vi "PPMS Interface_dev_IVdynamic.vi"() -> ()   [LabVIEW 2020]
uses:
  <vilib>/Analysis/1siggen.llb/Ramp Pattern by Samples.vi
  <vilib>/Utility/file.llb/Write Delimited Spreadsheet (string).vi
  <vilib>/Utility/file.llb/Write Delimited Spreadsheet (DBL).vi
  <vilib>/Analysis/NI_AALBase.lvlib
panel:
  in  "AC IV Path":path=path "C:/Users/QDUser/Desktop/LabVIEW Programs/PPMS Interface/lib/Measure IV AC.vi"
  out "IV Data":dbl[][](array[numeric])
  in  "DC IV Path":path=path "C:/Users/QDUser/Desktop/LabVIEW Programs/PPMS Interface/lib/Measure IV DC.vi"
  in  "scan_npts":i16
  out "scan_points":dbl[](array[numeric])
  out "scan_RATE":dbl=20.0
  out "scan_counter":i16=1000
  out "scan_head":i32=55
  out "scan_new":bool caption="Scan New"
  out "scan_env":string="MEASURE"
  out "Seq Line Now":i32=55
  out "AC Flag":bool caption="AC Current"
  in  "Filetype":u16(ring)=2 items=[".xlsx", ".txt", ".csv"]
  out "Wait Done":dbl=10.0
  in  "Measurement setup tabs":enum32{"DC Setup", "AC Setup", "I-V Setup"}(tab)=enum."AC Setup"
  in  "DC Pulse":bool=TRUE caption="Current Pulsing"
  in  "Channel 2":bool
  in  "Channel 1":bool=TRUE
  in  "Current Amplitude":string="1e-4"
  in  "Time Period (s)":string="3"
  in  "Tpad(ms)":i32=200
  in  "Voltmeter Range (V)":string="0.01"
  in  "NPLC":string="1"
  in  "Voltmeter Buffer Size":string="62"
  in  "Voltmeter 2 Address":string="8"
  in  "Voltmeter 1 Address":string="7"
  in  "6221 Address":string="12"
  in  "Configure DC System":bool
  in  "6221 Address 2":string="12" caption="6221 Address"
  in  "Current Amplitude 2":string="1e-4" caption="Current \nAmplitude"
  in  "Ch2 Enable":bool
  in  "Ch1 Enable":bool=TRUE
  in  "Buffer Data":enum16{"X", "XY", "RT", "XYRT"}(ring)=enum."RT"
  in  "Rate decimation":i32=2
  in  "SR860 Ch2 Address":string="5"
  in  "SR860 Ch1 Address":string="4"
  in  "Frequency":string="1711"
  in  "Filter BW":T1(ring)=enum."100ms"
  in  "Ch1 Harmonic":T2(ring)
  in  "Buffer Size (kB)":i32=2
  in  "Configure AC System":bool
  in  "Buffer Offset (kb)":string="0"
  in  "Ch2 Harmonic":T2(ring)
  in  "IV Datafile Root":path=path "C:/Users/QDUser/Desktop/LabVIEW Programs/PPMS External Control/testfiles/data/test_IV_file"
  in  "SR860 Address - IV":string="4" caption="SR860 Address"
  in  "6221 Address - IV":string="12" caption="6221 Address"
  in  "IV Sampling":enum16{"Linear", "Logartihmic"}(ring)=enum."Logartihmic"
  in  "IV Type":T3(ring)
  in  "dI or Imin":dbl=1e-08
  in  "Imax":dbl=0.0001
  in  "Points":i16=17
  in  "2182A Address - IV":string="7" caption="2182A Address"
  in  "IV - DC/AC":bool=TRUE
  in  "DC Period (s)":string="0.5" caption="6221 Address"
  in  "2182A Buffer":string="11" caption="6221 Address"
  in  "Ch1 Harmonic - IV":T2(ring) caption="Harmonic"
  in  "Frequency - IV":string="1711" caption="Frequency"
  in  "Filter BW - IV":T4(ring)=enum."10 ms" caption="Filter BW"
  in  "Measurement \nSetup":u16(ring)=1 items=["DC Setup", "AC Setup", "I-V Setup"]
  in  "Measure Device":bool caption="Measure \nDevice"
  in  "Y-axis":u16(ring)=6 items=["Serial Number", "Time Elapsed (s)", "Temperature (K)", "Field (Oe)", "Theta (degree)", "Current excitation (A)", "Resistance 1 (ohm)", "STD 1 (ohm)", "Resistance 2 (ohm)", "STD 2 (ohm)"]
  in  "X-axis":u16(ring)=1 items=["Serial Number", "Time Elapsed (s)", "Temperature (K)", "Field (Oe)", "Theta (degree)", "Current excitation (A)", "Resistance 1 (ohm)", "STD 1 (ohm)", "Resistance 2 (ohm)", "STD 2 (ohm)"]
  out "XY Graph":cluster{"Data array":dbl[], "Data array":dbl[]}(graph)={"Data array"=[1000.1076049804688, 1000.095458984375, 1000.1318969726562, 999.822021484375, 916.6700439453125, 830.8634643554688, 742.8192749023438, 654.9420776367188, 567.0899047851562, 479.1545104980469, 392.864013671875, 304.93212890625, 216.95523071289062, 129.0848846435547, 41.132198333740234, -44.77364730834961, -132.77415466308594, -218.81509399414062, -306.63739013671875, -394.50677490234375, -482.4195251464844, -570.4457397460938, -658.3638305664062, -744.2162475585938, -832.0615234375, -920.28857421875, -999.9136352539062, -999.8893432617188, -999.877197265625, -966.5936279296875, -880.3653564453125, -790.4647827148438, -704.466064453125, -616.628173828125, -528.7174682617188, -442.6363525390625, -352.7901916503906, -266.7317810058594, -178.9671173095703, -91.0753402709961, -3.042452096939087, 84.87220001220703, 170.94114685058594, 258.7779235839844, 346.6785583496094, 434.949462890625, 520.9051513671875, 608.9139404296875, 696.776611328125, 782.679931640625, 870.5813598632812, 958.4483642578125, 1000.1197509765625, 1000.095458984375], "Data array"=[2.0974435134090905, 2.0958316086363635, 2.0992071125, 2.0990977595454545, 2.107740888863636, 2.1053484827272726, 2.1082263649999997, 2.1037182222727275, 2.083242016590909, 2.081601890227273, 2.0829138438636363, 2.0798880874999996, 2.0791002761363635, 2.0677500127272728, 1.8619974204545455, 1.1222847387045454, 0.8201078938409091, 0.7255154414090907, 0.6976336516363636, 0.7003691852045455, 0.6927557248181818, 0.7014058921818181, 0.6990065759090907, 0.7079667083181819, 0.7010926857727272, 0.6957325292954544, 0.6955325533636365, 0.697872530181818, 0.711508848840909, 0.7229268473181818, 0.7067185125454545, 0.6959014081136364, 0.6962725788181818, 0.7031570712499998, 0.6892584726363638, 0.6798120112272727, 0.6948854190227274, 0.70866324875, 0.7220332009318181, 0.7281562234318182, 1.006325211, 1.7135642684090908, 1.949954792045455, 2.0590681531818182, 2.084260665, 2.087814913863636, 2.0882882709090906, 2.090093333181818, 2.0964560554545457, 2.1017757368181815, 2.103902046363636, 2.0958079104545453, 2.1060686974999996, 2.0965902061363635]}
  out "WAIT delay(s)":u32=10
  out "Data array":dbl[][](array[numeric])=[[1.0, 6.770192623138428, 299.99371337890625, -0.21726149320602417, 1.5735626220703125e-05, 0.0001, 2.778791197215469, 4.9368163008028935e-05, 0.24972602368222852, 0.020281499748667414], [2.0, 7.491643905639648, 299.9942932128906, -0.18105125427246094, 1.5735626220703125e-05, 0.0001, 2.778727154009175, 6.4560265668386335e-06, 0.24972602368222852, 0.020281499748667414], [3.0, 8.487261295318604, 299.9942932128906, -0.1689811646938324, 1.5735626220703125e-05, 0.0001, 2.778744486704454, 1.7432909608260873e-05, 0.24972602368222852, 0.020281499748667414], [4.0, 9.48760461807251, 299.9942932128906, -0.13277092576026917, 1.5735626220703125e-05, 0.0001, 2.7787373721821496, 1.0546280876721618e-05, 0.24972602368222852, 0.020281499748667414], [5.0, 10.486587047576904, 299.9942932128906, -0.18105125427246094, 1.5735626220703125e-05, 0.0001, 2.7787324108885514, 3.3140482153642334e-05, 0.24972602368222852, 0.020281499748667414], [6.0, 11.4936203956604, 299.9934997558594, -0.18105125427246094, 1.5735626220703125e-05, 0.0001, 2.7787128306044906, 8.738452653686467e-06, 0.24972602368222852, 0.020281499748667414], [7.0, 12.49498462677002, 299.9945068359375, -0.19312132894992828, 1.5735626220703125e-05, 0.0001, 2.778717373530526, 1.2274295922687026e-05, 0.24972602368222852, 0.020281499748667414], [8.0, 13.48988676071167, 299.9934997558594, -0.13277092576026917, 1.5735626220703125e-05, 0.0001, 2.7787547378466115, 1.0476339631891657e-05, 0.24972602368222852, 0.020281499748667414], [9.0, 14.494624614715576, 299.99468994140625, -0.18105125427246094, 1.5735626220703125e-05, 0.0001, 2.778750005063557, 1.3525812875041782e-05, 0.24972602368222852, 0.020281499748667414], [10.0, 15.49260950088501, 299.9933166503906, -0.18105125427246094, 1.5735626220703125e-05, 0.0001, 2.7787062629158754, 2.7302146994026072e-05, 0.24972602368222852, 0.020281499748667414], [11.0, 16.499380588531494, 299.99371337890625, -0.15691107511520386, 1.5735626220703125e-05, 0.0001, 2.7787572696524876, 4.561674974874875e-06, 0.24972602368222852, 0.020281499748667414], [12.0, 17.49661350250244, 299.9934997558594, -0.18105125427246094, 1.5735626220703125e-05, 0.0001, 2.7787224780695396, 6.570900725445805e-06, 0.24972602368222852, 0.020281499748667414], [13.0, 18.497665405273438, 299.9945068359375, -0.1448410004377365, 1.5735626220703125e-05, 0.0001, 2.7787587305283523, 5.038803697902784e-06, 0.24972602368222852, 0.020281499748667414], [14.0, 19.49858045578003, 299.9950866699219, -0.15691107511520386, 1.5735626220703125e-05, 0.0001, 2.7787560520664556, 2.3516873520935964e-05, 0.24972602368222852, 0.020281499748667414], [15.0, 20.502262115478516, 299.9945068359375, -0.1689811646938324, 1.5735626220703125e-05, 0.0001, 2.778759658212948, 1.0146691047534865e-05, 0.24972602368222852, 0.020281499748667414], [16.0, 21.509231090545654, 299.9933166503906, -0.1448410004377365, 1.5735626220703125e-05, 0.0001, 2.778762108164301, 1.6415144776984754e-05, 0.24972602368222852, 0.020281499748667414], [17.0, 22.504271984100342, 299.99468994140625, -0.1448410004377365, 1.5735626220703125e-05, 0.0001, 2.7787481940322323, 2.1730261379125438e-06, 0.24972602368222852, 0.020281499748667414], [18.0, 23.50353240966797, 299.9956970214844, -0.18105125427246094, 1.5735626220703125e-05, 0.0001, 2.7786632040260884, 4.100489486033837e-06, 0.24972602368222852, 0.020281499748667414], [19.0, 24.50387668609619, 299.9950866699219, -0.13277092576026917, 1.5735626220703125e-05, 0.0001, 2.7786751718394953, 1.5029701767803034e-05, 0.24972602368222852, 0.020281499748667414], [20.0, 25.50730562210083, 299.9950866699219, -0.12070083618164062, 1.5735626220703125e-05, 0.0001, 2.778733916102283, 7.323185001950876e-06, 0.24972602368222852, 0.020281499748667414], [21.0, 26.509282112121582, 299.99530029296875, -0.13277092576026917, 1.5735626220703125e-05, 0.0001, 2.778727512122714, 1.5472384423108354e-05, 0.24972602368222852, 0.020281499748667414], [22.0, 27.50660276412964, 299.99468994140625, -0.1448410004377365, 1.5735626220703125e-05, 0.0001, 2.7786470684532105, 5.001628372356291e-06, 0.24972602368222852, 0.020281499748667414], [23.0, 28.508782863616943, 299.9950866699219, -0.1689811646938324, 1.5735626220703125e-05, 0.0001, 2.7787105375409737, 1.5109466664788739e-05, 0.24972602368222852, 0.020281499748667414]]
  out "Time Elasped":dbl format="%#_13g"
  out "Serial Number":i32=23
  out "Current StartTime":timestamp=timestamp(3802691718.054652 s since 1904-01-01)
  out "Current Filename":path=path "C:/Users/qmgmit/Desktop/Shivam/data/FGaT-WTe2/20230715_FGaT-WTe2_chip3_D1/test_sweep_0715_1929.csv"
  in  "Metadata":string="***** Metadata *****\nSample Description: Dummy\nCreator: Shivam\n"
  out "SET Rate":dbl=20.0
  out "SET Setpoint":dbl=1000.0
  out "Current Line Number":i32=10
  out "Parameters":dbl[][](array[numeric])
  out "ENV VAR":string="MEASURE"
  out "Current Line":string="STOP MEASURE "
  out "Command":string="STOP"
  in  "Datafile Path":path=path "C:/Users/QDUser/Desktop/LabVIEW Programs/PPMS External Control/testfiles/data/test_datafile_00_0602_1858.txt"
  out "Line Count":i32=10
  out "Array of commands":string[][](array[string])=[["## Field sweep to test device health"], ["NEWFILE test_sweep"], [""], ["START MEASURE"], ["WAIT MEASURE 10"], ["SET FIELD -1000 RATE 20"], ["WAIT FIELD 10"], ["SET FIELD 1000 RATE 20"], ["WAIT FIELD 10"], ["STOP MEASURE "]]
  out "Sequence File":string="## Field sweep to test device health\nNEWFILE test_sweep\n\nSTART MEASURE\nWAIT MEASURE 10\nSET FIELD -1000 RATE 20\nWAIT FIELD 10\nSET FIELD 1000 RATE 20\nWAIT FIELD 10\nSTOP MEASURE "
  in  "Sequence File":path=path "C:/Users/QDUser/Desktop/LabVIEW Programs/PPMS External Control/testfiles/seq/test_seq.lseq"
  out "STOP Flag":bool=TRUE
  out "Measure Blink":bool
  in  "Stop sequence":bool
  in  "Start Sequence":bool caption="Set Temperature"
  out "ExecSeq":bool caption="Executing Sequence"
  out "Measure Flag":bool caption="Measurement in progress"
  out "Field\nStatus":i32(ring)=4 items=["MagnetUnknown"=0, "StablePersistent"=1, "WarmingSwitch"=2, "CoolingSwitch"=3, "StableDriven"=4, "Iterating"=5, "Charging"=6, "Discharging"=7, "CurrentError"=8, "MagnetFailure"=15]
  out "Temperature\nStatus":i32(ring)=1 items=["TemperatureUnknown"=0, "Stable"=1, "Tracking"=2, "Near"=5, "Chasing"=6, "Filling"=7, "Standby"=10, "Disabled"=13, "ImpedanceNotFunction"=14, "TempFailure"=15]
  out "Chamber\nStatus":i32(ring)=1 items=["ChamberUnknown"=0, "PurgedAndSealed"=1, "VentedAndSealed"=2, "Sealed"=3, "Purging"=4, "Venting"=5, "PreHiVac"=6, "HighVac"=7, "PumpContinuous"=8, "VentContinuous"=9, "ChamberFailure"=15]
  out "Initialised":bool=TRUE
  in  "STOP Button":bool=TRUE
  in  "Set Chamber":bool caption="Set Temperature"
  in  "Set Position":bool caption="Set Temperature"
  in  "Set Field":bool caption="Set Temperature"
  in  "Set Temperature":bool
  in  "Chamber Setpoint":i32(ring)=5 caption="Chamber" items=["Seal", "PurgeAndSeal", "VentAndSeal", "PumpContinuous", "VentContinuous", "HighVacuum"]
  out "Theta":dbl=1.5735626220703125e-05 caption="Position"
  in  "Theta Setpoint":dbl caption="Theta (degrees)" min=-10.0 max=370.0
  out "Field":dbl=-0.10863074660301208
  out "Temperature":dbl=299.9990539550781
  in  "Field Setpoint":dbl=1000.0 caption="Field (Oe)" min=-90000.0 max=90000.0
  in  "Temperature setpoint":dbl=300.0 caption="Temperature (K)" min=1.8 max=400.0
  in  "InstrumentType":i32(ring)=2 items=["PPMS", "VersaLab", "DynaCool", "SVSM", "OptiCool"]
  in  "Remote \nMode":bool
  in  "IP Address":string="10.29.168.8"
  # "AC IV"
  # "DC IV"
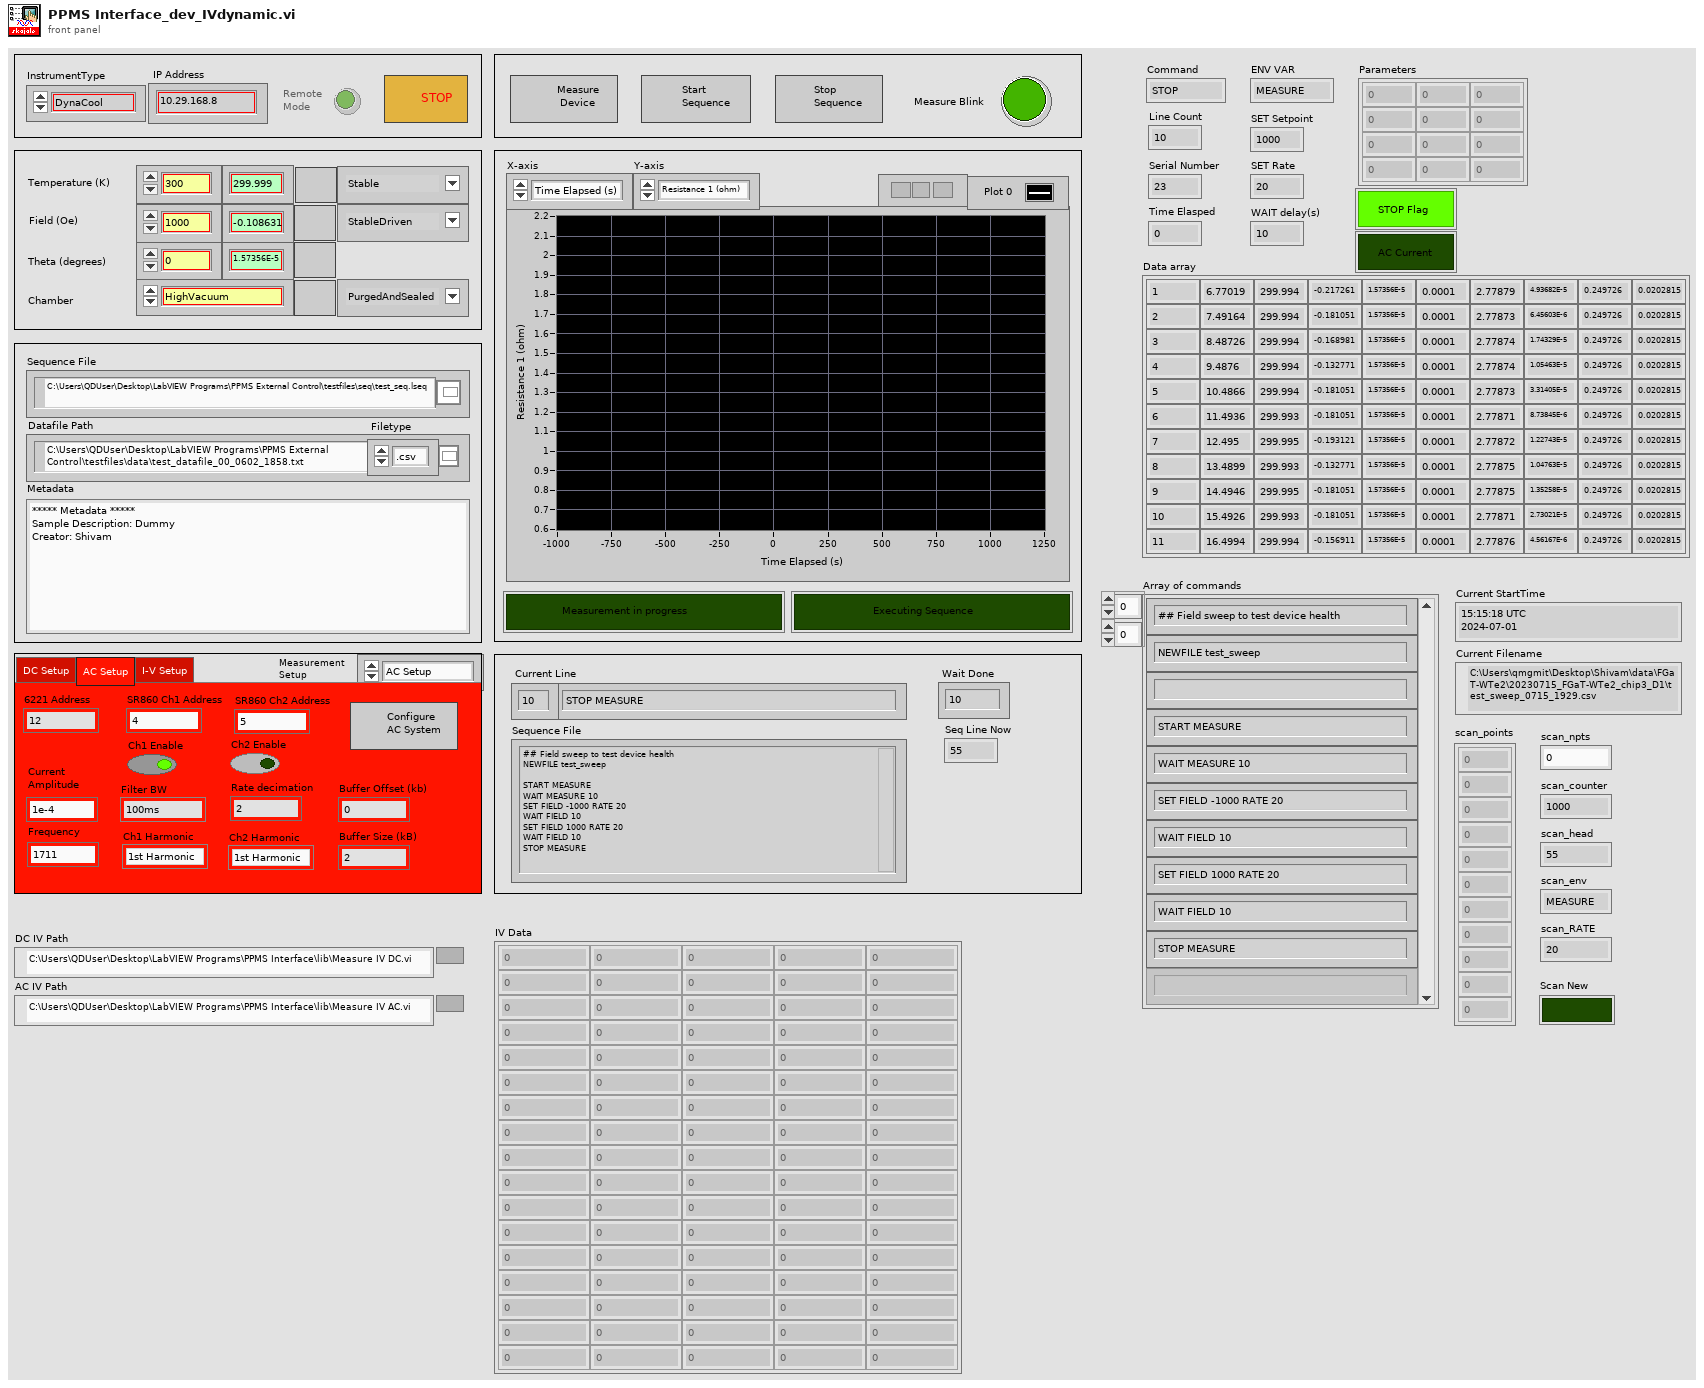
[diagram p1: front panel]
types:
  T1 = enum16{"1us", "3us", "10us", "30us", "100us", "300us", "1ms", "3ms", "10ms", "30ms", "100ms", "300ms", "1s"}
  T2 = enum16{"1st Harmonic", "2nd Harmonic", "3rd Harmonic"}
  T3 = enum16{"0 : Imax", "0 : Imax : 0", "0 : Imax : -Imax : 0"}
  T4 = enum16{"1 us", "3 us", "10 us", "30 us", "100 us", "300 us", "1 ms", "3 ms", "10 ms", "30 ms", "100 ms", "300 ms", "1 s", "3 s", "10 s", "30 s", "100 s", "300 s"}
  T5 = enum32{"Bad", "Idle", "Run top level", "Running"}
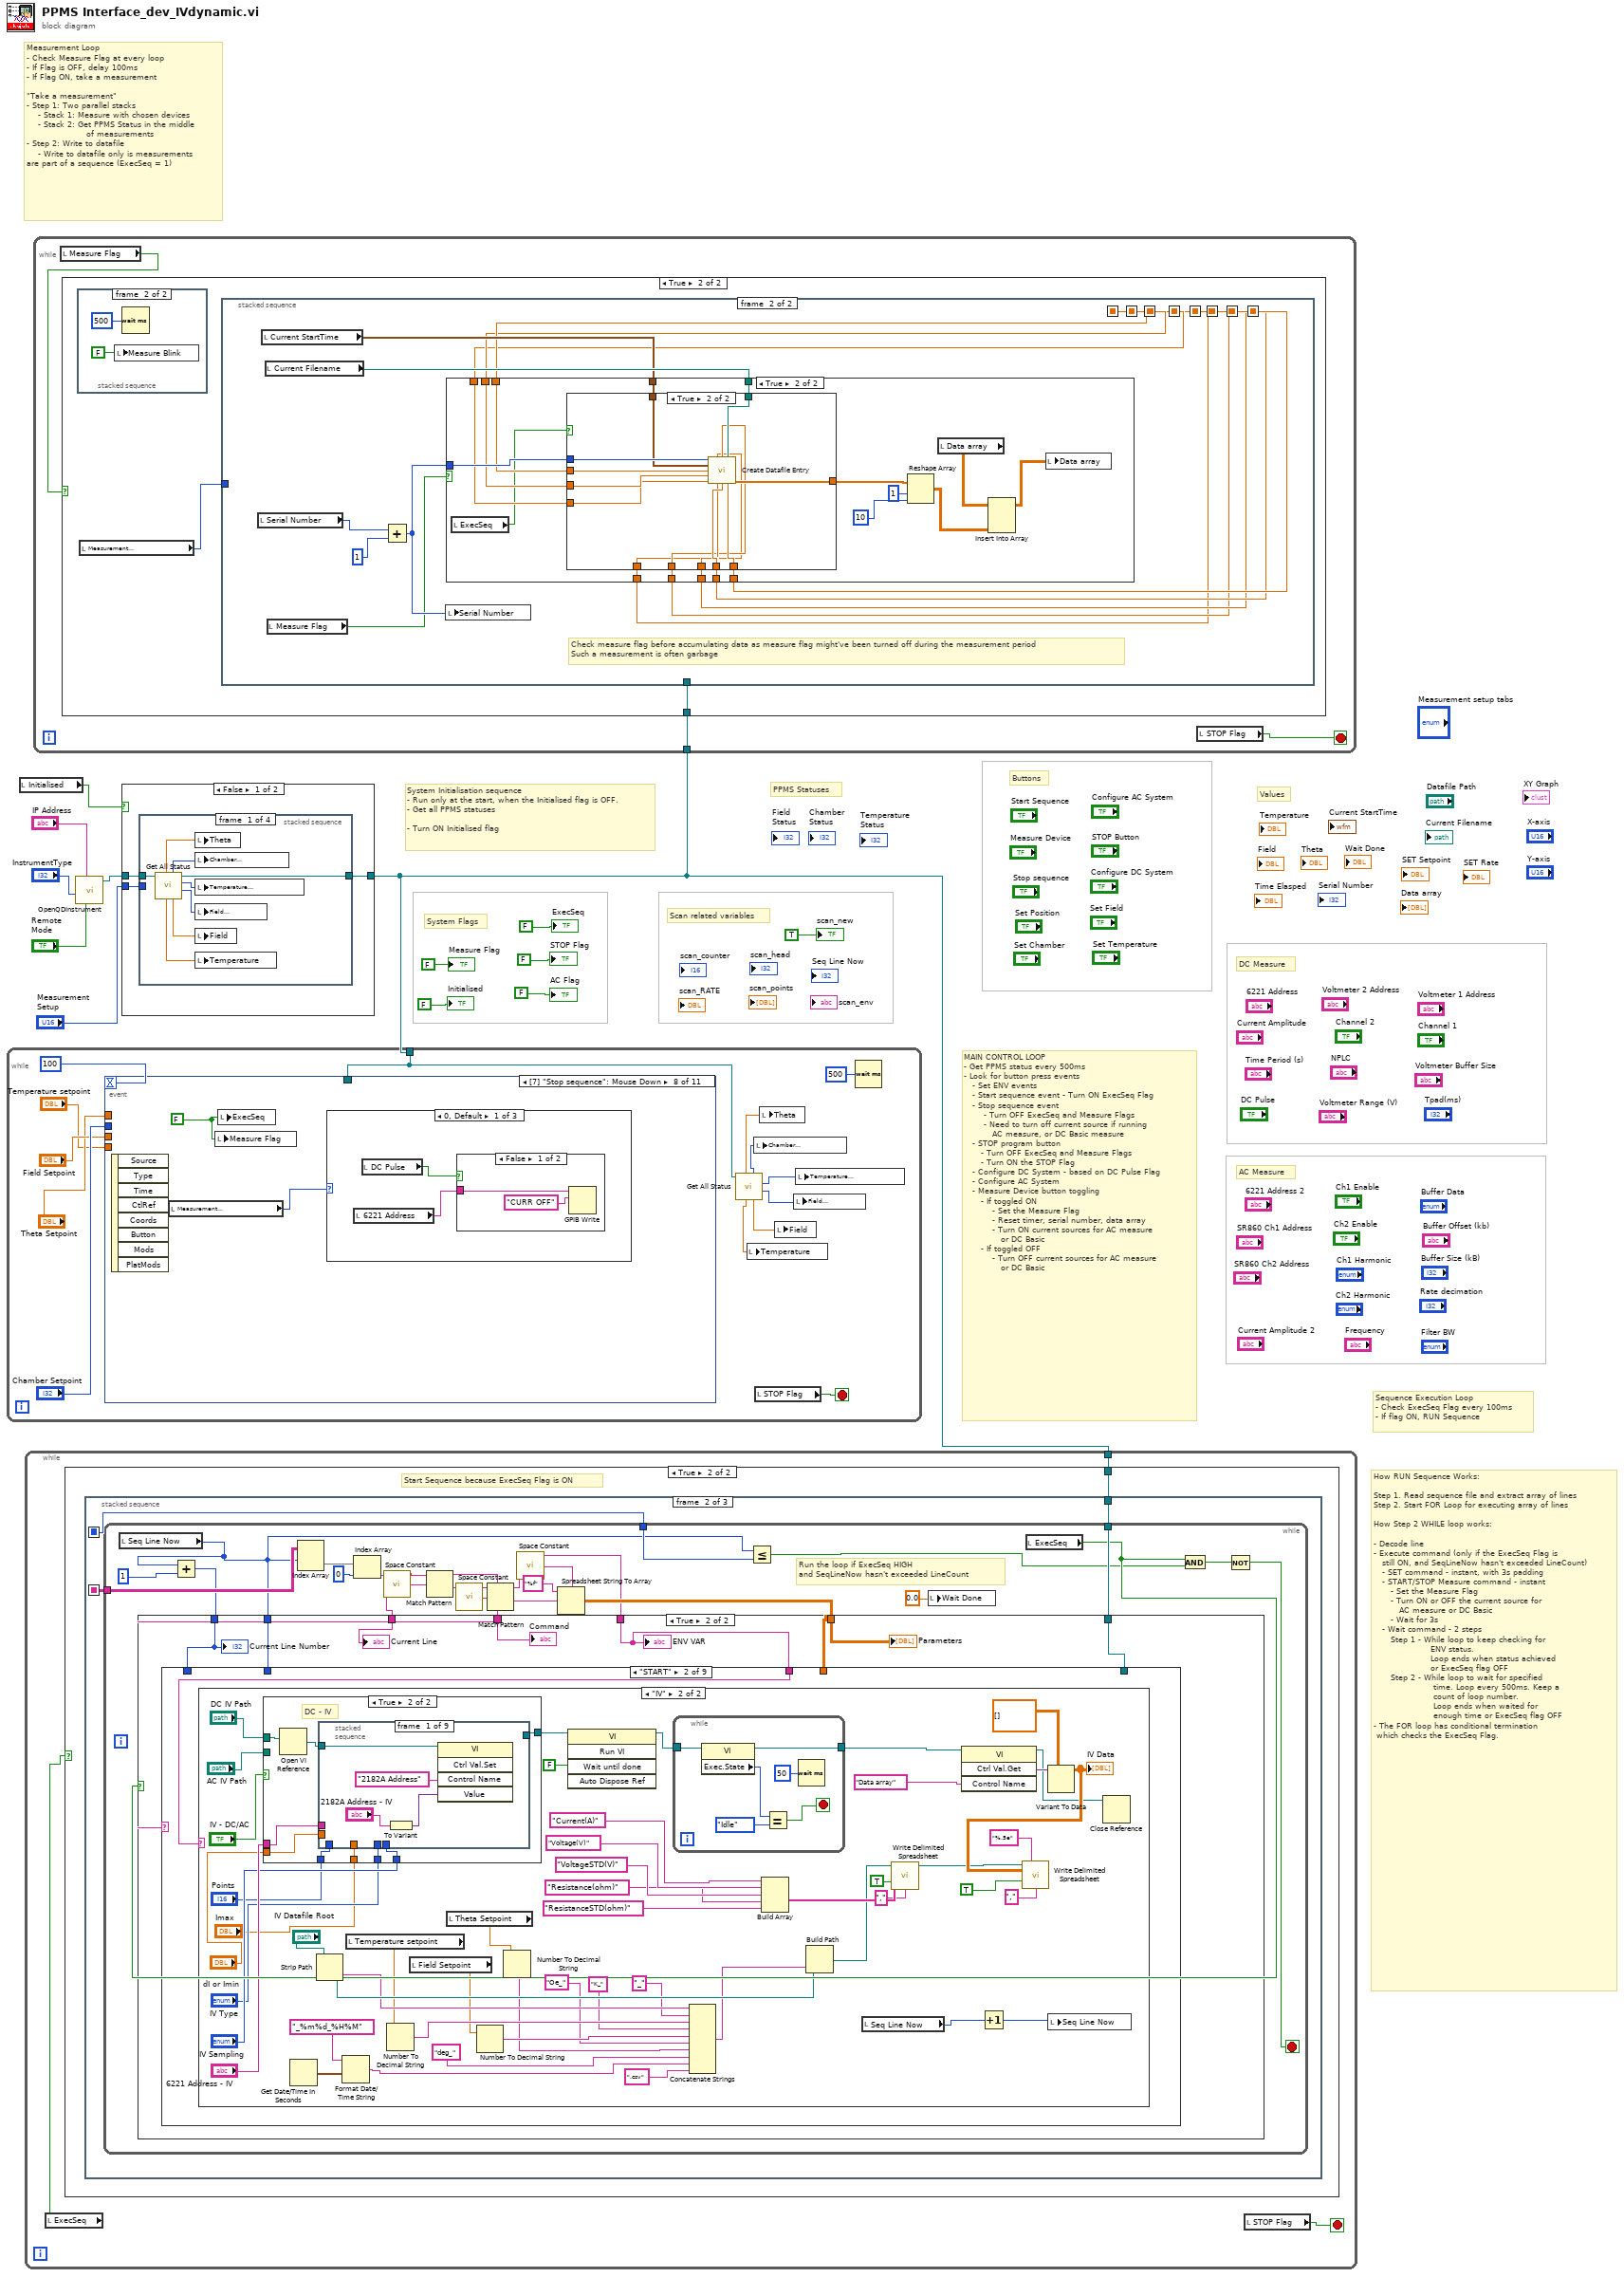
[diagram p0: block diagram]
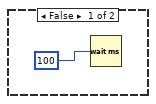
[diagram p2: hidden frame]
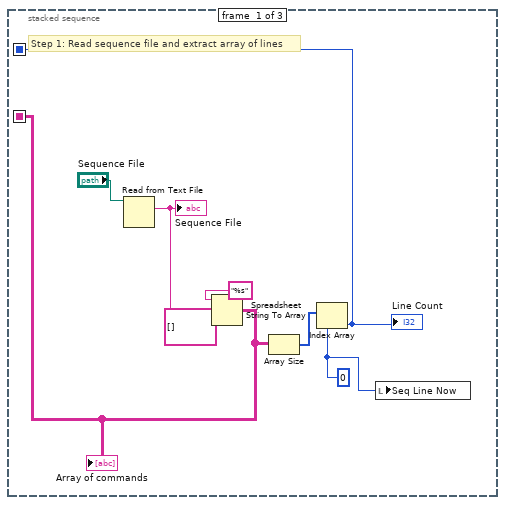
[diagram p3: hidden frame]
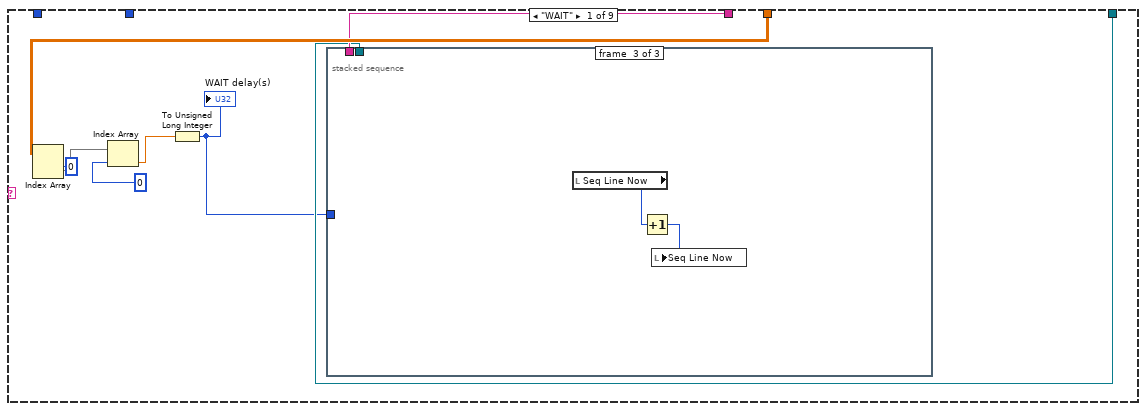
[diagram p5: hidden frame]
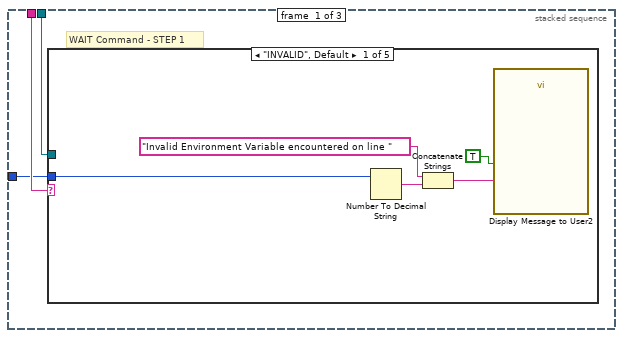
[diagram p6: hidden frame]
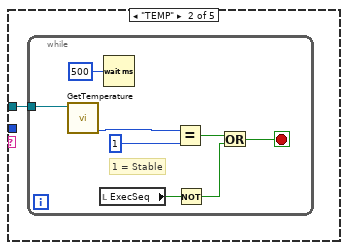
[diagram p7: hidden frame]
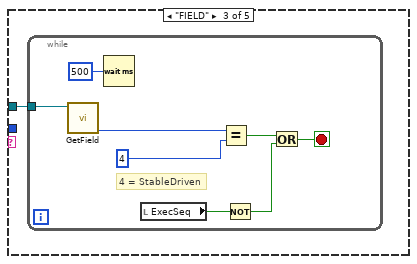
[diagram p8: hidden frame]
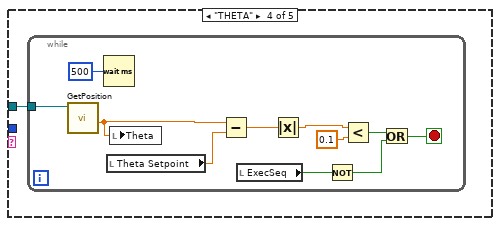
[diagram p9: hidden frame]
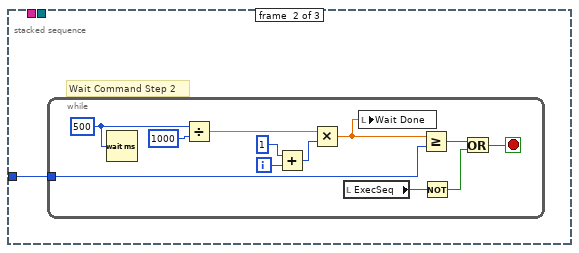
[diagram p11: hidden frame]
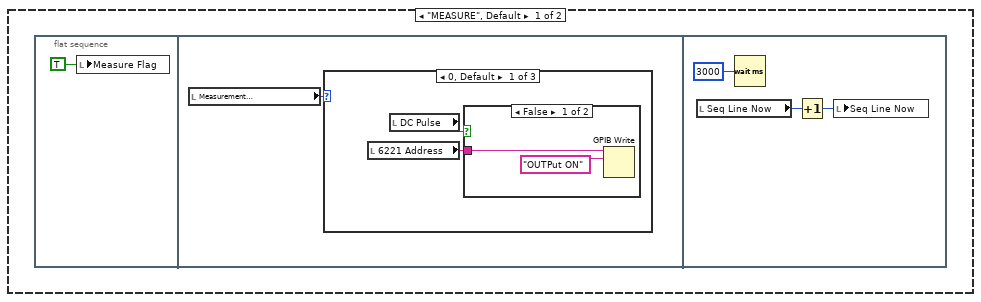
[diagram p12: hidden frame]
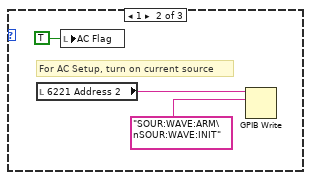
[diagram p14: hidden frame]
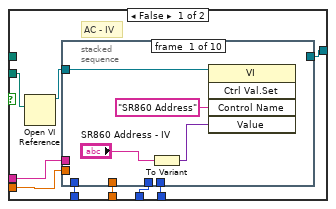
[diagram p16: hidden frame]
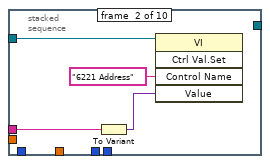
[diagram p17: hidden frame]
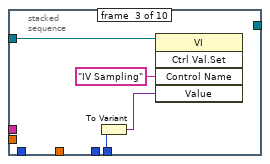
[diagram p18: hidden frame]
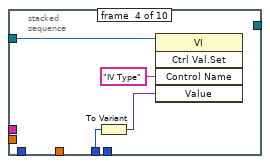
[diagram p19: hidden frame]
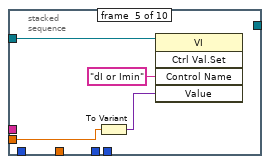
[diagram p20: hidden frame]
diagram:
  # "Scan related variables"
  # "AC Measure"
  # "DC Measure"
  # "How RUN Sequence Works:\n\nStep 1. Read sequence file and extract array of lines \nStep 2. Start FOR Loop for executing array of lines\n\nHow Step 2 WHILE loop works:\n\n- Decode line\n- Execute command (only if the ExecSeq Flag is \n   still ON, and SeqLineNow hasn't exceeded LineCount)\n   - SET command - instant, with 3s padding\n   - START/STOP Measure command - instant\n      - Set the Measure Flag\n      - Turn ON or OFF the current source for \n         AC measure or DC Basic\n      - Wait for 3s\n   - Wait command - 2 steps\n      Step 1 - While loop to keep checking for\n                    ENV status.\n                    Loop ends when status achieved \n                    or ExecSeq flag OFF\n      Step 2 - While loop to wait for specified \n                     time. Loop every 500ms. Keep a \n                     count of loop number.\n                     Loop ends when waited for \n                     enough time or ExecSeq flag OFF\n- The FOR loop has conditional termination\n which checks the ExecSeq Flag."
  # "Sequence Execution Loop\n- Check ExecSeq Flag every 100ms\n- If flag ON, RUN Sequence"
  # "MAIN CONTROL LOOP\n- Get PPMS status every 500ms\n- Look for button press events\n   - Set ENV events\n   - Start sequence event - Turn ON ExecSeq Flag\n   - Stop sequence event \n       - Turn OFF ExecSeq and Measure Flags\n       - Need to turn off current source if running\n          AC measure, or DC Basic measure\n   - STOP program button \n      - Turn OFF ExecSeq and Measure Flags\n      - Turn ON the STOP Flag\n   - Configure DC System - based on DC Pulse Flag\n   - Configure AC System\n   - Measure Device button toggling\n      - If toggled ON \n          - Set the Measure Flag\n          - Reset timer, serial number, data array\n          - Turn ON current sources for AC measure \n             or DC Basic\n      - If toggled OFF\n          - Turn OFF current sources for AC measure \n             or DC Basic"
  # "System Flags"
  # "PPMS Statuses"
  # "Values"
  # "Buttons"
  # "System Initialisation sequence\n- Run only at the start, when the Initialised flag is OFF.\n- Get all PPMS statuses\n\n- Turn ON Initialised flag"
  # "Measurement Loop\n- Check Measure Flag at every loop\n- If Flag is OFF, delay 100ms\n- If Flag ON, take a measurement\n\n\"Take a measurement\"\n- Step 1: Two parallel stacks\n    - Stack 1: Measure with chosen devices\n    - Stack 2: Get PPMS Status in the middle\n                     of measurements\n- Step 2: Write to datafile\n    - Write to datafile only is measurements    are part of a sequence (ExecSeq = 1)"
  n1 = local read "Initialised"() -> (w9:bool)
  n2 = call "OpenQDInstrument.vi"("Remote"="Remote \nMode", "IP Address"="IP Address", "InstrumentType"="InstrumentType") -> ("Instrument Ref"=w8:refnum<k24>)  [unwired: 5 in, 1 out]
  n3 = case shown="False" w9 {
    tunnel: w8 -> [w16 w27]
    tunnel: [w15 w27] -> w4
    tunnel: "Measurement \nSetup" -> [w14 _]
    frame False {
      n4 = stacked-sequence {
        tunnel: w16 -> [w24 _ _ _]
        tunnel: [w18 _ _ _] -> w15
        tunnel: w14 -> [_ _ _ _]
        frame #0 {
          n5 = call "Get All Status.vi"("Instrument Ref In"=w24) -> ("Field\nStatus"=w21:i32, "Temperature\nStatus"=w22:i32, "Instrument Ref Out"=w18:refnum<k24>, "Field"=w19:dbl, "Chamber\nStatus"=w23:i32, "Temperature"=w20:dbl, "Position"=w17:dbl)  [unwired: 3 in, 1 out]
          n6 = local write "Theta"(w17) -> ()
          n7 = local write "Chamber\nStatus"(w23) -> ()
          n8 = local write "Temperature\nStatus"(w22) -> ()
          n9 = local write "Field\nStatus"(w21) -> ()
          n10 = local write "Field"(w19) -> ()
          n11 = local write "Temperature"(w20) -> ()
        }
        frame #1 {
          n12 = Wait (ms)(milliseconds to wait=u32 100) -> ()  [unwired: 1 out]
        }
        frame #2 {
        }
        frame #3 {
          n13 = local write "Initialised"(TRUE ("Initialised")) -> ()
        }
      }
    }
    frame True {
    }
  }
  n14 = while {
    tunnel: w4 -> [w32]
    stop <- w29 stop-if-true
    n15 = event shown="[7] \"Stop sequence\": Mouse Down" {
      selector: _ -> [_ _ _ _ _ _ _ _ _ _ _]
      dyn-events: _ -> [_ _ _ _ _ _ _ _ _ _ _]
      timeout: 100 -> [_ _ _ _ _ _ _ _ _ _ _]
      tunnel: "Chamber Setpoint" -> [_ _ w73 _ _ _ _ _ _ _ _]
      tunnel: w32 -> [_ _ w72 w77 w79 w83 _ _ _ _ _]
      tunnel: "Temperature setpoint" -> [_ _ _ w74 _ _ _ _ _ _ _]
      tunnel: "Field Setpoint" -> [_ _ _ _ w78 _ _ _ _ _ _]
      tunnel: "Theta Setpoint" -> [_ _ _ _ _ w82 _ _ _ _ _]
      event Timeout {
        # "Use timeout to update graph"
        n16 = event-data() -> ()  [unwired: 1 in, 3 out]
        n17 = local read "Data array"() -> (w49:dbl[][])
        n18 = property on="Y-axis" class="Ring (strict)"() -> ("RingText.Text"=w42:string)  [unwired: 2 in, 2 out]
        n19 = property on="X-axis" class="Ring (strict)"() -> ("RingText.Text"=w43:string)  [unwired: 2 in, 2 out]
        n20 = local read "Y-axis"() -> (w45:u16)
        n21 = local read "X-axis"() -> (w46:u16)
        n22 = Index Array(array=w49, index (col) #1=w46, index (col) #2=w45) -> (element #1=w48:dbl[], element #2=w47:dbl[])  [unwired: 2 in]
        n23 = Bundle("Data array"=w48, "Data array"=w47) -> (w44:cluster{"Data array":dbl[], "Data array":dbl[]})  [unwired: 1 in]
        n24 = property on="XY Graph" class="XYGraph (strict)"("XScale.NameLbl.Text"=w43, "YScale.NameLbl.Text"=w42) -> ()  [unwired: 2 in, 2 out]
        n25 = local write "XY Graph"(w44) -> ()
      }
      event "Measure Device": Value Change {
        n26 = event-data() -> ()  [unwired: 1 in, 6 out]
        n27 = local read "Measure Device"() -> (w50:bool)
        n28 = case shown="True" w50 {
          frame False {
            n29 = local read "Measurement \nSetup"() -> (w51:u16)
            n30 = case shown="0, Default" w51 {
              frame 0, Default {
                # "Turn off 6221 if DC Basic"
                n31 = local read "6221 Address"() -> (w52:string)
                n32 = local read "DC Pulse"() -> (w53:bool)
                n33 = case shown="False" w53 {
                  tunnel: w52 -> [w54 _]
                  frame False {
                    n34 = GPIB Write(0:w54, 1:"OUTPut OFF" ("data")) -> ()  [unwired: 3 in, 2 out]
                  }
                  frame True {
                  }
                }
              }
              frame 1 {
                # "Turn off 6221 for AC System"
                n35 = local read "6221 Address 2"() -> (w56:string)
                n36 = GPIB Write(0:w56, 1:"SOUR:WAVE:ABORt" ("data")) -> ()  [unwired: 3 in, 2 out]
              }
              frame 2 {
              }
            }
          }
          frame True {
            n37 = Get Date/Time In Seconds() -> (seconds since 1Jan1904=w59:timestamp)
            n38 = local write "Time Elasped"(0.0 ("Time Elasped")) -> ()
            n39 = local write "Serial Number"(0 ("Serial Number")) -> ()
            n40 = local read "Measurement \nSetup"() -> (w58:u16)
            n41 = local write "Current StartTime"(w59) -> ()
            n42 = local write "Data array"(dbl[][] [] ("Data array")) -> ()
            n43 = case shown="0, Default" w58 {
              frame 0, Default {
                n44 = local read "6221 Address"() -> (w63:string)
                n45 = local read "DC Pulse"() -> (w64:bool)
                n46 = case shown="False" w64 {
                  tunnel: w63 -> [w66 _]
                  frame False {
                    n47 = Wait (ms)(milliseconds to wait=u32 1000) -> ()  [unwired: 1 out]
                    n48 = GPIB Write(0:w66, 1:"OUTPut ON" ("data")) -> ()  [unwired: 3 in, 2 out]
                  }
                  frame True {
                  }
                }
              }
              frame 1 {
                n49 = local read "6221 Address 2"() -> (w70:string)
                n50 = local write "AC Flag"(TRUE ("AC Flag")) -> ()
                n51 = Wait (ms)(milliseconds to wait=u32 1000) -> ()  [unwired: 1 out]
                n52 = GPIB Write(0:w70, 1:"SOUR:WAVE:ARM\nSOUR:WAVE:INIT" ("data")) -> ()  [unwired: 3 in, 2 out]
              }
              frame 2 {
              }
            }
          }
        }
        n53 = local write "Measure Flag"(w50) -> ()
      }
      event "Set Chamber": Mouse Down {
        n54 = event-data() -> ()  [unwired: 1 in, 8 out]
        n55 = call "SetChamber.vi"("Code"=w73, "Instrument Ref In"=w72) -> ()  [unwired: 1 in, 3 out]
      }
      event "Set Temperature": Mouse Down {
        w75 = 0 items=["FastSettle", "NoOvershoot"] ("Approach")
        n56 = event-data() -> ()  [unwired: 1 in, 8 out]
        n57 = call "SetTemperature.vi"("Approach"=w75, "Rate"=10.0, "Temperature"=w74, "Instrument Ref In"=w77) -> ()  [unwired: 3 in, 3 out]
      }
      event "Set Field": Mouse Down {
        n58 = event-data() -> ()  [unwired: 1 in, 8 out]
        n59 = call "SetField.vi"("Rate"=200.0, "Field"=w78, "Instrument Ref In"=w79) -> ()  [unwired: 4 in, 3 out]
      }
      event "Set Position": Mouse Down {
        n60 = event-data() -> ()  [unwired: 1 in, 8 out]
        n61 = call "SetPosition.vi"("Speed"=2.0, "Position"=w82, "Instrument Ref In"=w83) -> ()  [unwired: 4 in, 3 out]
      }
      event "Start Sequence": Mouse Down {
        n62 = event-data() -> ()  [unwired: 1 in, 8 out]
        n63 = local write "ExecSeq"(TRUE ("ExecSeq")) -> ()
      }
      event "Stop sequence": Mouse Down {
        w86 = FALSE ("ExecSeq")
        n64 = event-data() -> ()  [unwired: 1 in, 8 out]
        n65 = local read "Measurement \nSetup"() -> (w85:u16)
        n66 = local write "Measure Flag"(w86) -> ()
        n67 = local write "ExecSeq"(w86) -> ()
        n68 = case shown="0, Default" w85 {
          frame 0, Default {
            n69 = local read "6221 Address"() -> (w87:string)
            n70 = local read "DC Pulse"() -> (w88:bool)
            n71 = case shown="False" w88 {
              tunnel: w87 -> [w89 _]
              frame False {
                n72 = GPIB Write(0:w89, 1:"CURR OFF" ("data")) -> ()  [unwired: 3 in, 2 out]
              }
              frame True {
              }
            }
          }
          frame 1 {
            n73 = local read "6221 Address 2"() -> (w92:string)
            n74 = GPIB Write(0:w92, 1:"SOUR:WAVE:ABORt" ("data")) -> ()  [unwired: 3 in, 2 out]
          }
          frame 2 {
          }
        }
      }
      event "STOP Button": Mouse Down {
        n75 = event-data() -> ()  [unwired: 1 in, 8 out]
        n76 = stacked-sequence {
          frame #0 {
            w93 = FALSE ("Measure Flag")
            n77 = local write "ExecSeq"(w93) -> ()
            n78 = local write "Measure Flag"(w93) -> ()
          }
          frame #1 {
            n79 = Wait (ms)(milliseconds to wait=u32 1000) -> ()  [unwired: 1 out]
          }
          frame #2 {
            n80 = local write "STOP Flag"(TRUE ("STOP Flag")) -> ()
          }
        }
      }
      event "Configure DC System": Mouse Down {
        n81 = event-data() -> ()  [unwired: 1 in, 8 out]
        n82 = local read "Current Amplitude"() -> (w97:string)
        n83 = local read "Time Period (s)"() -> (w98:string)
        n84 = local read "6221 Address"() -> (w103:string)
        n85 = local read "Voltmeter Range (V)"() -> (w100:string)
        n86 = local read "NPLC"() -> (w99:string)
        n87 = local read "Voltmeter 1 Address"() -> (w104:string)
        n88 = local read "Voltmeter Buffer Size"() -> (w101:string)
        n89 = local read "Channel 2"() -> (w102:bool)
        n90 = local read "Voltmeter 2 Address"() -> (w105:string)
        n91 = local read "DC Pulse"() -> (w96:bool)
        n92 = local read "Channel 1"() -> (w106:bool)
        n93 = case shown="True" w96 {
          tunnel: w106 -> [w115 w125]
          tunnel: w105 -> [w114 w124]
          tunnel: w104 -> [w113 w123]
          tunnel: w103 -> [w112 w122]
          tunnel: w102 -> [w108 w121]
          tunnel: w101 -> [w107 w120]
          tunnel: w100 -> [w109 w119]
          tunnel: w99 -> [w110 w118]
          tunnel: w98 -> [_ w117]
          tunnel: w97 -> [w111 w116]
          frame False {
            n94 = call "DC Basic Configure.vi"("Channel 2"=w108, "Channel 1"=w115, "Voltmeter Buffer Size"=w107, "Voltmeter 2 Address"=w114, "Voltmeter Range (V)"=w109, "Voltmeter 1 Address"=w113, "NPLC"=w110, "Current Amplitude"=w111, "6221 Address"=w112) -> ()  [unwired: 3 in]
          }
          frame True {
            n95 = call "DC Transport Configure.vi"("Channel 2"=w121, "Channel 1"=w125, "Voltmeter Buffer Size"=w120, "Voltmeter 2 Address"=w124, "Voltmeter Range (V)"=w119, "Voltmeter 1 Address"=w123, "NPLC"=w118, "Time Period (s)"=w117, "Current Amplitude"=w116, "6221 Address"=w122) -> ()  [unwired: 2 in]
          }
        }
      }
      event "Configure AC System": Mouse Down {
        n96 = event-data() -> ()  [unwired: 1 in, 8 out]
        n97 = local read "SR860 Ch1 Address"() -> (w132:string)
        n98 = local read "Current Amplitude 2"() -> (w134:string)
        n99 = local read "Buffer Size (kB)"() -> (w128:i32)
        n100 = local read "Ch1 Harmonic"() -> (w127:T2)
        n101 = local read "Frequency"() -> (w135:string)
        n102 = local read "Filter BW"() -> (w136:T1)
        n103 = local read "6221 Address 2"() -> (w133:string)
        n104 = local read "Ch2 Harmonic"() -> (w126:T2)
        n105 = local read "Ch1 Enable"() -> (w131:bool)
        n106 = local read "SR860 Ch2 Address"() -> (w130:string)
        n107 = local read "Rate decimation"() -> (w137:i32)
        n108 = local read "Ch2 Enable"() -> (w129:bool)
        n109 = call "AC Transport Configure.vi"("6221 Address"=w133, "SR860 Ch1 Address"=w132, "Ch1 Enable"=w131, "SR860 Ch2 Address"=w130, "Ch2 Enable"=w129, "Current Amplitude"=w134, "Frequency"=w135, "Filter BW"=w136, "Buffer Size (kB)"=w128, "Ch1 Harmonic"=w127, "Ch2 Harmonic"=w126, "Rate decimation"=w137) -> ()  [unwired: 1 in, 3 out]
      }
    }
    n110 = call "Get All Status.vi"("Instrument Ref In"=w32) -> ("Field\nStatus"=w36:i32, "Temperature\nStatus"=w35:i32, "Field"=w38:dbl, "Chamber\nStatus"=w34:i32, "Temperature"=w37:dbl, "Position"=w31:dbl)  [unwired: 3 in, 2 out]
    n111 = local write "Temperature"(w37) -> ()
    n112 = local write "Chamber\nStatus"(w34) -> ()
    n113 = local read "STOP Flag"() -> (w29:bool)
    n114 = local write "Theta"(w31) -> ()
    n115 = local write "Field"(w38) -> ()
    n116 = local write "Field\nStatus"(w36) -> ()
    n117 = local write "Temperature\nStatus"(w35) -> ()
    n118 = Wait (ms)(milliseconds to wait=u32 500) -> ()  [unwired: 1 out]
  }
  n119 = while {
    tunnel: w4 -> [w138]
    stop <- w140 stop-if-true
    n120 = local read "ExecSeq"() -> (w139:bool)
    n121 = case shown="True" w139 {
      tunnel: w138 -> [_ w142]
      frame False {
        n122 = Wait (ms)(milliseconds to wait=u32 100) -> ()  [unwired: 1 out]
      }
      frame True {
        # "Start Sequence because ExecSeq Flag is ON"
        n123 = stacked-sequence {
          seq-local: [w145 _ _] -> [_ w151 _]
          seq-local: [w144 _ _] -> [_ w153 _]
          tunnel: w142 -> [_ w152 _]
          frame #0 {
            w143 = 0 ("index")
            # "Step 1: Read sequence file and extract array of lines"
            n124 = Read from Text File(file (use dialog)="Sequence File") -> (text=w149:string)  [unwired: 3 in, 3 out]
            "Sequence File" <- w149
            n125 = Spreadsheet String To Array(format string="%s", spreadsheet string=w149, array type (2D Dbl)=string[][] []) -> (array=w144:string[][])  [unwired: 1 in]
            "Array of commands" <- w144
            n126 = Array Size(array=w144) -> (size(s)=w150:i32[])
            n127 = Index Array(array=w150, index=w143) -> (element=w145:i32)
            "Line Count" <- w145
            n128 = local write "Seq Line Now"(w143) -> ()
          }
          frame #1 {
            n129 = while {
              tunnel: w153 -> [w168]
              tunnel: w152 -> [w162]
              tunnel: w151 -> [w158]
              stop <- w161 stop-if-true
              # "Run the loop if ExecSeq HIGH\nand SeqLineNow hasn't exceeded LineCount"
              n130 = local read "Seq Line Now"() -> (w154:i32)
              n131 = Add(x=w154, y=1) -> (x+y=w160:i32)
              n132 = Index Array(array=w168, index (row)=w154) -> (element=w167:string[])  [unwired: 1 in]
              n133 = Index Array(array=w167, index=0) -> (element=w166:string)
              n134 = call <vilib>:"Space Constant.vi"() -> ("String"=w176:string)
              n135 = Match Pattern(string=w166, regular expression=w176) -> (before substring=w165:string, after substring=w174:string)  [unwired: 1 in, 2 out]
              n136 = call <vilib>:"Space Constant.vi"() -> ("String"=w173:string)
              n137 = Match Pattern(string=w174, regular expression=w173) -> (before substring=w163:string, after substring=w171:string)  [unwired: 1 in, 2 out]
              n138 = call <vilib>:"Space Constant.vi"() -> ("String"=w170:string)
              n139 = Spreadsheet String To Array(delimiter (Tab)=w170, format string="%f", spreadsheet string=w171) -> (array=w164:dbl[][])  [unwired: 1 in]
              n140 = Less Or Equal?(x=w154, y=w158) -> (x <= y?=w155:bool)
              n141 = local write "Wait Done"(0.0 ("Wait Done")) -> ()
              n142 = local read "ExecSeq"() -> (w156:bool)
              n143 = case shown="True" w156 {
                tunnel: w166 -> [_ w183]
                tunnel: w165 -> [_ w182]
                tunnel: w164 -> [_ w181]
                tunnel: w163 -> [_ w180]
                tunnel: w162 -> [_ w179]
                tunnel: w160 -> [_ w178]
                tunnel: w154 -> [_ w177]
                frame False {
                }
                frame True {
                  n144 = case shown="\"START\"" w182 {
                    tunnel: w181 -> [w187 _ _ w425 w504 _ _ _ w539]
                    tunnel: w180 -> [w186 w245 _ w424 _ w524 _ _ w536]
                    tunnel: w178 -> [_ _ _ w422 _ _ _ _ w535]
                    tunnel: w179 -> [w185 _ _ w423 _ _ _ _ w534]
                    tunnel: w177 -> [_ _ _ w426 _ _ _ _ _]
                    frame "WAIT" {
                      n145 = Index Array(array=w187, index (row)=0) -> (element=w188:dbl[])  [unwired: 1 in]
                      n146 = Index Array(array=w188, index=0) -> (element=w189:dbl)
                      n147 = To Unsigned Long Integer(number=w189) -> (unsigned 32bit integer=w184:u32)
                      "WAIT delay(s)" <- w184
                      n148 = stacked-sequence {
                        tunnel: w186 -> [w194 _ _]
                        tunnel: w184 -> [w193 w230 _]
                        tunnel: w185 -> [w192 _ _]
                        frame #0 {
                          # "WAIT Command - STEP 1"
                          n149 = case shown="\"INVALID\", Default" w194 {
                            tunnel: w193 -> [w196 _ _ _ _]
                            tunnel: w192 -> [_ w200 w209 w218 _]
                            frame "INVALID", Default {
                              n150 = Number To Decimal String(number=w196) -> (decimal integer string=w197:string)  [unwired: 1 in]
                              n151 = Concatenate Strings("Invalid Environment Variable encountered on line " ("string"), w197) -> (w195:string)
                              n152 = call "Display Message to User2"("Enable"=TRUE, "Message"=w195) -> ()  [unwired: 8 in, 2 out]
                            }
                            frame "TEMP" {
                              n153 = while {
                                tunnel: w200 -> [w201]
                                stop <- w202 stop-if-true
                                # "1 = Stable"
                                n154 = call "GetTemperature.vi"("Instrument Ref In"=w201) -> ("Temperature\nStatus"=w206:i32)  [unwired: 4 in, 4 out]
                                n155 = local read "ExecSeq"() -> (w205:bool)
                                n156 = Wait (ms)(milliseconds to wait=u32 500) -> ()  [unwired: 1 out]
                                n157 = Equal?(x=w206, y=1) -> (x = y?=w204:bool)
                                n158 = Not(x=w205) -> (.not. x?=w203:bool)
                                n159 = Or(x=w204, y=w203) -> (x .or. y?=w202:bool)
                              }
                            }
                            frame "FIELD" {
                              n160 = while {
                                tunnel: w209 -> [w211]
                                stop <- w212 stop-if-true
                                # "4 = StableDriven"
                                n161 = call "GetField.vi"("Instrument Ref In"=w211) -> ("Field\nStatus"=w215:i32)  [unwired: 4 in, 4 out]
                                n162 = Wait (ms)(milliseconds to wait=u32 500) -> ()  [unwired: 1 out]
                                n163 = local read "ExecSeq"() -> (w214:bool)
                                n164 = Equal?(x=w215, y=4) -> (x = y?=w213:bool)
                                n165 = Not(x=w214) -> (.not. x?=w210:bool)
                                n166 = Or(x=w213, y=w210) -> (x .or. y?=w212:bool)
                              }
                            }
                            frame "THETA" {
                              n167 = while {
                                tunnel: w218 -> [w224]
                                stop <- w219 stop-if-true
                                n168 = call "GetPosition.vi"("Instrument Ref In"=w224) -> ("Position"=w228:dbl)  [unwired: 3 in, 3 out]
                                n169 = Wait (ms)(milliseconds to wait=u32 500) -> ()  [unwired: 1 out]
                                n170 = local read "Theta Setpoint"() -> (w223:dbl)
                                n171 = local write "Theta"(w228) -> ()
                                n172 = Subtract(x=w228, y=w223) -> (x-y=w227:dbl)
                                n173 = local read "ExecSeq"() -> (w222:bool)
                                n174 = Absolute Value(x=w227) -> (abs(x)=w226:dbl)
                                n175 = Not(x=w222) -> (.not. x?=w221:bool)
                                n176 = Less?(x=w226, y=0.1) -> (x < y?=w220:bool)
                                n177 = Or(x=w220, y=w221) -> (x .or. y?=w219:bool)
                              }
                            }
                            frame "MEASURE" {
                            }
                          }
                        }
                        frame #1 {
                          # "Wait Command Step 2"
                          n178 = while {
                            tunnel: w230 -> [w232]
                            i -> [w241]
                            stop <- w236 stop-if-true
                            w240 = u32 500 ("milliseconds to wait")
                            n179 = Wait (ms)(milliseconds to wait=w240) -> ()  [unwired: 1 out]
                            n180 = Divide(x=w240, y=u32 1000) -> (x/y=w238:dbl)
                            n181 = Add(x=1, y=w241) -> (x+y=w234:i32)
                            n182 = Multiply(x=w238, y=w234) -> (x*y=w231:dbl)
                            n183 = local read "ExecSeq"() -> (w242:bool)
                            n184 = local write "Wait Done"(w231) -> ()
                            n185 = Greater Or Equal?(x=w231, y=w232) -> (x >= y?=w237:bool)
                            n186 = Not(x=w242) -> (.not. x?=w235:bool)
                            n187 = Or(x=w237, y=w235) -> (x .or. y?=w236:bool)
                          }
                        }
                        frame #2 {
                          n188 = local read "Seq Line Now"() -> (w243:i32)
                          n189 = Increment(x=w243) -> (x+1=w244:i32)
                          n190 = local write "Seq Line Now"(w244) -> ()
                        }
                      }
                    }
                    frame "START" {
                      n191 = case shown="\"IV\"" w245 {
                        frame "MEASURE", Default {
                          n192 = flat-sequence {
                            frame #0 {
                              n193 = local write "Measure Flag"(TRUE ("Measure Flag")) -> ()
                            }
                            frame #1 {
                              n194 = local read "Measurement \nSetup"() -> (w247:u16)
                              n195 = case shown="0, Default" w247 {
                                frame 0, Default {
                                n196 = local read "6221 Address"() -> (w248:string)
                                n197 = local read "DC Pulse"() -> (w249:bool)
                                n198 = case shown="False" w249 {
                                tunnel: w248 -> [w250 _]
                                frame False {
                                n199 = GPIB Write(0:w250, 1:"OUTPut ON" ("data")) -> ()  [unwired: 3 in, 2 out]
                                }
                                frame True {
                                }
                                }
                                }
                                frame 1 {
                                # "For AC Setup, turn on current source"
                                n200 = local read "6221 Address 2"() -> (w254:string)
                                n201 = local write "AC Flag"(TRUE ("AC Flag")) -> ()
                                n202 = GPIB Write(0:w254, 1:"SOUR:WAVE:ARM\nSOUR:WAVE:INIT" ("data")) -> ()  [unwired: 3 in, 2 out]
                                }
                                frame 2 {
                                }
                              }
                            }
                            frame #2 {
                              n203 = local read "Seq Line Now"() -> (w255:i32)
                              n204 = Wait (ms)(milliseconds to wait=u32 3000) -> ()  [unwired: 1 out]
                              n205 = Increment(x=w255) -> (x+1=w256:i32)
                              n206 = local write "Seq Line Now"(w256) -> ()
                            }
                          }
                        }
                        frame "IV" {
                          n207 = case shown="True" "IV - DC/AC" {
                            tunnel: [w317 w367] -> w308
                            tunnel: "DC IV Path" -> [_ w365]
                            tunnel: "AC IV Path" -> [w316 _]
                            tunnel: "6221 Address - IV" -> [w314 w364]
                            tunnel: "IV Sampling" -> [w313 w363]
                            tunnel: "IV Type" -> [w312 w362]
                            tunnel: "dI or Imin" -> [w311 w361]
                            tunnel: "Imax" -> [w310 w360]
                            tunnel: "Points" -> [w309 w359]
                            frame False {
                              # "AC - IV"
                              n208 = Open VI Reference(vi path=w316) -> (vi reference=w315:refnum<vi>)  [unwired: 5 in, 1 out]
                              n209 = stacked-sequence {
                                tunnel: [_ _ _ _ _ _ _ _ _ w354] -> w317
                                tunnel: w315 -> [w318 w323 w327 w331 w335 w339 w343 w346 w350 w355]
                                tunnel: w314 -> [_ w322 _ _ _ _ _ _ _ _]
                                tunnel: w313 -> [_ _ w326 _ _ _ _ _ _ _]
                                tunnel: w312 -> [_ _ _ w330 _ _ _ _ _ _]
                                tunnel: w311 -> [_ _ _ _ w334 _ _ _ _ _]
                                tunnel: w310 -> [_ _ _ _ _ w338 _ _ _ _]
                                tunnel: w309 -> [_ _ _ _ _ _ w342 _ _ _]
                                frame #0 {
                                n210 = To Variant(anything="SR860 Address - IV") -> (Variant=w320:variant)
                                n211 = invoke class="VI" method="Ctrl Val.Set"(reference=w318, "Control Name"="SR860 Address", "Value"=w320) -> ()  [unwired: 2 in, 5 out]
                                }
                                frame #1 {
                                n212 = To Variant(anything=w322) -> (Variant=w324:variant)
                                n213 = invoke class="VI" method="Ctrl Val.Set"(reference=w323, "Control Name"="6221 Address", "Value"=w324) -> ()  [unwired: 2 in, 5 out]
                                }
                                frame #2 {
                                n214 = To Variant(anything=w326) -> (Variant=w328:variant)
                                n215 = invoke class="VI" method="Ctrl Val.Set"(reference=w327, "Control Name"="IV Sampling", "Value"=w328) -> ()  [unwired: 2 in, 5 out]
                                }
                                frame #3 {
                                n216 = To Variant(anything=w330) -> (Variant=w332:variant)
                                n217 = invoke class="VI" method="Ctrl Val.Set"(reference=w331, "Control Name"="IV Type", "Value"=w332) -> ()  [unwired: 2 in, 5 out]
                                }
                                frame #4 {
                                n218 = To Variant(anything=w334) -> (Variant=w336:variant)
                                n219 = invoke class="VI" method="Ctrl Val.Set"(reference=w335, "Control Name"="dI or Imin", "Value"=w336) -> ()  [unwired: 2 in, 5 out]
                                }
                                frame #5 {
                                n220 = To Variant(anything=w338) -> (Variant=w340:variant)
                                n221 = invoke class="VI" method="Ctrl Val.Set"(reference=w339, "Control Name"="Imax", "Value"=w340) -> ()  [unwired: 2 in, 5 out]
                                }
                                frame #6 {
                                n222 = To Variant(anything=w342) -> (Variant=w344:variant)
                                n223 = invoke class="VI" method="Ctrl Val.Set"(reference=w343, "Control Name"="Ipts", "Value"=w344) -> ()  [unwired: 2 in, 5 out]
                                }
                                frame #7 {
                                n224 = To Variant(anything="Frequency - IV") -> (Variant=w348:variant)
                                n225 = invoke class="VI" method="Ctrl Val.Set"(reference=w346, "Control Name"="Frequency", "Value"=w348) -> ()  [unwired: 2 in, 5 out]
                                }
                                frame #8 {
                                n226 = To Variant(anything="Filter BW - IV") -> (Variant=w352:variant)
                                n227 = invoke class="VI" method="Ctrl Val.Set"(reference=w350, "Control Name"="Filter BW", "Value"=w352) -> ()  [unwired: 2 in, 5 out]
                                }
                                frame #9 {
                                n228 = To Variant(anything="Ch1 Harmonic - IV") -> (Variant=w357:variant)
                                n229 = invoke class="VI" method="Ctrl Val.Set"(reference=w355, "Control Name"="Ch1 Harmonic", "Value"=w357) -> (reference out=w354:refnum<vi>)  [unwired: 2 in, 4 out]
                                }
                              }
                            }
                            frame True {
                              # "DC - IV"
                              n230 = Open VI Reference(vi path=w365) -> (vi reference=w366:refnum<vi>)  [unwired: 5 in, 1 out]
                              n231 = stacked-sequence {
                                tunnel: w366 -> [w371 w375 w379 w383 w387 w391 w395 w399 w404]
                                tunnel: [_ _ _ _ _ _ _ _ w400] -> w367
                                tunnel: w364 -> [_ w372 _ _ _ _ _ _ _]
                                tunnel: w363 -> [_ _ w376 _ _ _ _ _ _]
                                tunnel: w362 -> [_ _ _ w380 _ _ _ _ _]
                                tunnel: w361 -> [_ _ _ _ w384 _ _ _ _]
                                tunnel: w360 -> [_ _ _ _ _ w388 _ _ _]
                                tunnel: w359 -> [_ _ _ _ _ _ w392 _ _]
                                frame #0 {
                                n232 = To Variant(anything="2182A Address - IV") -> (Variant=w369:variant)
                                n233 = invoke class="VI" method="Ctrl Val.Set"(reference=w371, "Control Name"="2182A Address", "Value"=w369) -> ()  [unwired: 2 in, 5 out]
                                }
                                frame #1 {
                                n234 = To Variant(anything=w372) -> (Variant=w373:variant)
                                n235 = invoke class="VI" method="Ctrl Val.Set"(reference=w375, "Control Name"="6221 Address", "Value"=w373) -> ()  [unwired: 2 in, 5 out]
                                }
                                frame #2 {
                                n236 = To Variant(anything=w376) -> (Variant=w377:variant)
                                n237 = invoke class="VI" method="Ctrl Val.Set"(reference=w379, "Control Name"="IV Sampling", "Value"=w377) -> ()  [unwired: 2 in, 5 out]
                                }
                                frame #3 {
                                n238 = To Variant(anything=w380) -> (Variant=w381:variant)
                                n239 = invoke class="VI" method="Ctrl Val.Set"(reference=w383, "Control Name"="IV Type", "Value"=w381) -> ()  [unwired: 2 in, 5 out]
                                }
                                frame #4 {
                                n240 = To Variant(anything=w384) -> (Variant=w385:variant)
                                n241 = invoke class="VI" method="Ctrl Val.Set"(reference=w387, "Control Name"="dI or Imin", "Value"=w385) -> ()  [unwired: 2 in, 5 out]
                                }
                                frame #5 {
                                n242 = To Variant(anything=w388) -> (Variant=w389:variant)
                                n243 = invoke class="VI" method="Ctrl Val.Set"(reference=w391, "Control Name"="Imax", "Value"=w389) -> ()  [unwired: 2 in, 5 out]
                                }
                                frame #6 {
                                n244 = To Variant(anything=w392) -> (Variant=w393:variant)
                                n245 = invoke class="VI" method="Ctrl Val.Set"(reference=w395, "Control Name"="Ipts", "Value"=w393) -> ()  [unwired: 2 in, 5 out]
                                }
                                frame #7 {
                                n246 = To Variant(anything="DC Period (s)") -> (Variant=w397:variant)
                                n247 = invoke class="VI" method="Ctrl Val.Set"(reference=w399, "Control Name"="Period (s)", "Value"=w397) -> ()  [unwired: 2 in, 5 out]
                                }
                                frame #8 {
                                n248 = To Variant(anything="2182A Buffer") -> (Variant=w402:variant)
                                n249 = invoke class="VI" method="Ctrl Val.Set"(reference=w404, "Control Name"="2182A Buffer", "Value"=w402) -> (reference out=w400:refnum<vi>)  [unwired: 2 in, 4 out]
                                }
                              }
                            }
                          }
                          n250 = Get Date/Time In Seconds() -> (seconds since 1Jan1904=w270:timestamp)
                          n251 = Strip Path(path="IV Datafile Root") -> (stripped path=w293:path, name=w290:string)
                          n252 = Format Date/Time String(time format string (%c)="_%m%d_%H%M", seconds (now)=w270) -> (date/time string=w268:string)  [unwired: 1 in]
                          n253 = local read "Temperature setpoint"() -> (w288:dbl)
                          n254 = Number To Decimal String(number=w288) -> (decimal integer string=w287:string)  [unwired: 1 in]
                          n255 = local read "Field Setpoint"() -> (w285:dbl)
                          n256 = local read "Theta Setpoint"() -> (w282:dbl)
                          n257 = Number To Decimal String(number=w285) -> (decimal integer string=w284:string)  [unwired: 1 in]
                          n258 = Number To Decimal String(number=w282) -> (decimal integer string=w281:string)  [unwired: 1 in]
                          n259 = invoke class="VI" method="Run VI"(reference=w308, "Wait until done"=FALSE ("Wait Until Done")) -> (reference out=w302:refnum<vi>)  [unwired: 3 in, 4 out]
                          n260 = while {
                            tunnel: [w408] -> w303
                            tunnel: w302 -> [w407]
                            stop <- w406 stop-if-true
                            n261 = property class="VI"(reference=w407) -> (reference out=w408:refnum<vi>, "Exec.State"=w410:T5)  [unwired: 1 in, 1 out]
                            n262 = Equal?(x=w410, y=T5."Idle") -> (x = y?=w406:bool)
                            n263 = Wait (ms)(milliseconds to wait=u32 50) -> ()  [unwired: 1 out]
                          }
                          n264 = Concatenate Strings(w290, "_" ("string"), w287, "K_" ("string"), w284, "Oe_" ("string"), w281, "deg_" ("string"), w268, ".csv" ("string")) -> (w279:string)
                          n265 = Build Array("Current(A)", "Voltage(V)", "VoltageSTD(V)", "Resistance(ohm)", "ResistanceSTD(ohm)") -> (w301:string[])
                          n266 = Build Path(base path=w293, name or relative path=w279) -> (appended path=w292:path)
                          n267 = local read "Seq Line Now"() -> (w271:i32)
                          n268 = call-poly <vilib>:"Write Delimited Spreadsheet.vi"("file path (dialog if empty)"=w292, "1D data"=w301, "append to file? (new file:F)"=TRUE, "delimiter (\\t)"="," ("delimiter (\\t)")) -> ("new file path (Not A Path if cancelled)"=w274:path)  [unwired: 10 in, 1 out]
                          n269 = invoke class="VI" method="Ctrl Val.Get"(reference=w303, "Control Name"="Data array") -> (reference out=w273:refnum<vi>, "Get Control Value Variant"=w304:variant)  [unwired: 2 in, 2 out]
                          n270 = Increment(x=w271) -> (x+1=w272:i32)
                          n271 = Variant To Data(type=dbl[][] [] ("Data array"), Variant=w304) -> (data=w276:dbl[][])  [unwired: 1 in, 1 out]
                          "IV Data" <- w276
                          n272 = call-poly <vilib>:"Write Delimited Spreadsheet.vi"("file path (dialog if empty)"=w274, "format (%.3f)"="%.5e" ("format string"), "2D data"=w276, "append to file? (new file:F)"=TRUE, "delimiter (\\t)"="," ("delimiter (\\t)")) -> ()  [unwired: 9 in, 2 out]
                          n273 = local write "Seq Line Now"(w272) -> ()
                          n274 = Close Reference(reference=w273) -> ()  [unwired: 1 in, 1 out]
                        }
                      }
                    }
                    frame "STOP" {
                      n275 = flat-sequence {
                        frame #0 {
                          n276 = local write "Measure Flag"(FALSE ("Measure Flag")) -> ()
                        }
                        frame #1 {
                          n277 = local read "Measurement \nSetup"() -> (w412:u16)
                          n278 = case shown="2" w412 {
                            frame 0, Default {
                              n279 = local read "6221 Address"() -> (w413:string)
                              n280 = local read "DC Pulse"() -> (w414:bool)
                              n281 = case shown="False" w414 {
                                tunnel: w413 -> [w415 _]
                                frame False {
                                n282 = GPIB Write(0:w415, 1:"OUTPut OFF" ("data")) -> ()  [unwired: 3 in, 2 out]
                                }
                                frame True {
                                }
                              }
                            }
                            frame 1 {
                              # "Turn off current for AC System"
                              n283 = local read "6221 Address 2"() -> (w417:string)
                              n284 = GPIB Write(0:w417, 1:"SOUR:WAVE:ABORt" ("data")) -> ()  [unwired: 3 in, 2 out]
                            }
                            frame 2 {
                            }
                          }
                        }
                        frame #2 {
                          n285 = local read "Seq Line Now"() -> (w419:i32)
                          n286 = Wait (ms)(milliseconds to wait=u32 3000) -> ()  [unwired: 1 out]
                          n287 = Increment(x=w419) -> (x+1=w420:i32)
                          n288 = local write "Seq Line Now"(w420) -> ()
                        }
                      }
                    }
                    frame "SCAN" {
                      n289 = local read "scan_new"() -> (w427:bool)
                      n290 = case shown="False" w427 {
                        tunnel: w426 -> [_ w478]
                        tunnel: w425 -> [_ w477]
                        tunnel: w424 -> [_ w476]
                        tunnel: w423 -> [w431 _]
                        tunnel: w422 -> [w428 _]
                        frame False {
                          # "Not a new SCAN. Just go through the existing scan by setting the appropriate ENV"
                          n291 = local read "scan_points"() -> (w434:dbl[])
                          n292 = local read "scan_counter"() -> (w433:i16)
                          n293 = local read "scan_RATE"() -> (w430:dbl)
                          n294 = local read "scan_env"() -> (w429:string)
                          n295 = Index Array(array=w434, index=w433) -> (element=w432:dbl)
                          n296 = flat-sequence {
                            tunnel: w429 -> [w439]
                            tunnel: w428 -> [w438]
                            tunnel: w431 -> [w437]
                            tunnel: w432 -> [w436]
                            tunnel: w430 -> [w435]
                            frame #0 {
                              n297 = case shown="\"CURRENT\"" w439 {
                                tunnel: w438 -> [w440 _ _ _ _]
                                tunnel: w437 -> [_ w447 w450 w453 _]
                                tunnel: w436 -> [_ w445 w449 w452 w457]
                                tunnel: w435 -> [_ w446 w451 w454 _]
                                frame "INVALID", Default {
                                n298 = Number To Decimal String(number=w440) -> (decimal integer string=w442:string)  [unwired: 1 in]
                                n299 = Concatenate Strings("Invalid Environment Variable encountered on line " ("string"), w442) -> (w441:string)
                                n300 = call "Display Message to User3"("Enable"=TRUE, "Message"=w441) -> ()  [unwired: 8 in, 2 out]
                                }
                                frame "TEMP" {
                                w448 = 0 items=["FastSettle", "NoOvershoot"] ("Approach")
                                n301 = call "SetTemperature.vi"("Approach"=w448, "Rate"=w446, "Temperature"=w445, "Instrument Ref In"=w447) -> ()  [unwired: 3 in, 3 out]
                                n302 = local write "Temperature setpoint"(w445) -> ()
                                }
                                frame "FIELD" {
                                n303 = call "SetField.vi"("Rate"=w451, "Field"=w449, "Instrument Ref In"=w450) -> ()  [unwired: 4 in, 3 out]
                                n304 = local write "Field Setpoint"(w449) -> ()
                                }
                                frame "THETA" {
                                n305 = local write "Theta Setpoint"(w452) -> ()
                                n306 = call "SetPosition.vi"("Speed"=w454, "Position"=w452, "Instrument Ref In"=w453) -> ()  [unwired: 4 in, 3 out]
                                }
                                frame "CURRENT" {
                                n307 = local read "Measurement \nSetup"() -> (w455:u16)
                                n308 = Number To Exponential String(number=w457) -> (E-format string=w456:string)  [unwired: 3 in]
                                n309 = case shown="0, Default" w455 {
                                tunnel: w456 -> [w458 w469]
                                frame 0, Default {
                                n310 = local read "6221 Address"() -> (w460:string)
                                n311 = local write "Current Amplitude"(w458) -> ()
                                n312 = local read "DC Pulse"() -> (w459:bool)
                                n313 = case shown="True" w459 {
                                tunnel: w460 -> [w463 w466]
                                tunnel: w458 -> [w461 w467]
                                frame False {
                                n314 = Concatenate Strings("CURRent ", w461) -> (w462:string)
                                n315 = GPIB Write(0:w463, 1:w462) -> ()  [unwired: 3 in, 2 out]
                                }
                                frame True {
                                n316 = Concatenate Strings("SOUR:WAVE:AMPL " ("string"), w467) -> (w468:string)
                                n317 = GPIB Write(0:w466, 1:w468) -> ()  [unwired: 3 in, 2 out]
                                }
                                }
                                }
                                frame 1 {
                                n318 = local read "6221 Address 2"() -> (w470:string)
                                n319 = local write "Current Amplitude 2"(w469) -> ()
                                n320 = Concatenate Strings("SOUR:WAVE:AMPL " ("string"), w469) -> (w472:string)
                                n321 = GPIB Write(0:w470, 1:w472) -> ()  [unwired: 3 in, 2 out]
                                }
                                }
                                }
                              }
                            }
                            frame #1 {
                              n322 = local read "Seq Line Now"() -> (w473:i32)
                              n323 = Increment(x=w473) -> (x+1=w474:i32)
                              n324 = local write "Seq Line Now"(w474) -> ()
                              n325 = Wait (ms)(milliseconds to wait=u32 3000) -> ()  [unwired: 1 out]
                            }
                          }
                        }
                        frame True {
                          # "New SCAN just started"
                          n326 = flat-sequence {
                            tunnel: w478 -> [w480]
                            tunnel: w477 -> [w493]
                            tunnel: w476 -> [w482]
                            frame #0 {
                              n327 = local write "scan_head"(w480) -> ()
                              n328 = local write "scan_new"(FALSE ("scan_new")) -> ()
                            }
                            frame #1 {
                              w492 = 0 ("index (row)")
                              n329 = Index Array(array=w493, index (row)=w492) -> (element=w488:dbl[])  [unwired: 1 in]
                              n330 = Index Array(array=w493, index (row)=w492) -> (element=w489:dbl[])  [unwired: 1 in]
                              n331 = Index Array(array=w493, index (row)=w492) -> (element=w490:dbl[])  [unwired: 1 in]
                              n332 = Index Array(array=w493, index (row)=w492) -> (element=w491:dbl[])  [unwired: 1 in]
                              n333 = Index Array(array=w488, index=4) -> (element=w487:dbl)
                              n334 = Index Array(array=w489, index=2) -> (element=w481:dbl)
                              n335 = Index Array(array=w490, index=1) -> (element=w484:dbl)
                              n336 = Index Array(array=w491, index=0) -> (element=w485:dbl)
                              n337 = local write "scan_RATE"(w487) -> ()
                              n338 = local write "scan_npts"(w481) -> ()
                              n339 = call-poly <vilib>:"Ramp Pattern.vi"("exclude end?"=FALSE, "start"=w485, "end"=w484, "samples"=w481) -> ("Ramp Pattern"=w483:dbl[])  [unwired: 6 in, 1 out]
                              n340 = local write "scan_env"(w482) -> ()
                              n341 = local write "scan_points"(w483) -> ()
                            }
                            frame #2 {
                              n342 = local read "scan_head"() -> (w498:i32)
                              n343 = local write "Seq Line Now"(w498) -> ()
                              n344 = local write "scan_counter"(i16 0 ("scan_counter")) -> ()
                            }
                          }
                        }
                      }
                    }
                    frame "END" {
                      # "Check if SCAN endpoint reached"
                      n345 = Index Array(array=w504, index (row)=0) -> (element=w505:dbl[])  [unwired: 1 in]
                      n346 = local read "scan_counter"() -> (w503:i16)
                      n347 = Index Array(array=w505, index=2) -> ()  [unwired: 1 out]
                      n348 = Decrement(x="scan_npts") -> (x-1=w500:i16)
                      n349 = Less?(x=w503, y=w500) -> (x < y?=w501:bool)
                      n350 = case shown="False" w501 {
                        frame False {
                          # "SCAN endpoint reached.\nJust move SET the scan_new flag and move on to the next line"
                          n351 = local write "scan_new"(TRUE ("scan_new")) -> ()
                          n352 = local read "Seq Line Now"() -> (w509:i32)
                          n353 = Increment(x=w509) -> (x+1=w508:i32)
                          n354 = local write "Seq Line Now"(w508) -> ()
                        }
                        frame True {
                          # "Increment scan_counter\nChange SeqLineNow to scan_head"
                          # "SCAN endpoint not reached yet"
                          n355 = local read "scan_counter"() -> (w512:i16)
                          n356 = Increment(x=w512) -> (x+1=w513:i16)
                          n357 = local write "scan_counter"(w513) -> ()
                          n358 = local read "scan_head"() -> (w511:i32)
                          n359 = local write "Seq Line Now"(w511) -> ()
                        }
                      }
                    }
                    frame "NEWFILE" {
                      n360 = local read "Datafile Path"() -> (w526:path)
                      n361 = Strip Path(path=w526) -> (stripped path=w525:path)  [unwired: 1 out]
                      n362 = Build Path(base path=w525, name or relative path=w524) -> (appended path=w523:path)
                      n363 = local write "Datafile Path"(w523) -> ()
                      n364 = call "Create New Datafile.vi"("Metadata"="Metadata", "Filetype"="Filetype", "File Base"=w523) -> ("Start time"=w520:timestamp, "File name"=w521:path)
                      n365 = local write "Current Filename"(w521) -> ()
                      n366 = local write "Current StartTime"(w520) -> ()
                      n367 = local write "Time Elasped"(0.0 ("Time Elasped")) -> ()
                      n368 = local write "Serial Number"(0) -> ()
                      n369 = local write "Data array"(dbl[][] [] ("Data array")) -> ()
                      n370 = local read "Seq Line Now"() -> (w514:i32)
                      n371 = Increment(x=w514) -> (x+1=w515:i32)
                      n372 = local write "Seq Line Now"(w515) -> ()
                    }
                    frame "#", Default {
                      # "Let go. This is considered a comment"
                      n373 = local read "Seq Line Now"() -> (w527:i32)
                      n374 = Increment(x=w527) -> (x+1=w528:i32)
                      n375 = local write "Seq Line Now"(w528) -> ()
                    }
                    frame "" {
                      # "Blank line disregarded as a comment"
                      n376 = local read "Seq Line Now"() -> (w529:i32)
                      n377 = Increment(x=w529) -> (x+1=w530:i32)
                      n378 = local write "Seq Line Now"(w530) -> ()
                    }
                    frame "SET" {
                      n379 = Index Array(array=w539, index (row)=0) -> (element=w538:dbl[])  [unwired: 1 in]
                      n380 = Index Array(array=w539, index (row)=0) -> (element=w537:dbl[])  [unwired: 1 in]
                      n381 = Index Array(array=w538, index=0) -> (element=w533:dbl)
                      n382 = Index Array(array=w537, index=2) -> (element=w532:dbl)
                      n383 = local write "SET Rate"(w532) -> ()
                      n384 = local write "SET Setpoint"(w533) -> ()
                      n385 = flat-sequence {
                        tunnel: w536 -> [w547]
                        tunnel: w535 -> [w546]
                        tunnel: w534 -> [w545]
                        tunnel: w533 -> [w544]
                        tunnel: w532 -> [w543]
                        frame #0 {
                          n386 = case shown="\"CURRENT\"" w547 {
                            tunnel: w546 -> [w548 _ _ _ _]
                            tunnel: w545 -> [_ w555 w558 w561 _]
                            tunnel: w544 -> [_ w553 w557 w560 w565]
                            tunnel: w543 -> [_ w554 w559 w562 _]
                            frame "INVALID", Default {
                              n387 = Number To Decimal String(number=w548) -> (decimal integer string=w550:string)  [unwired: 1 in]
                              n388 = Concatenate Strings("Invalid Environment Variable encountered on line " ("string"), w550) -> (w549:string)
                              n389 = call "Display Message to User"("Enable"=TRUE, "Message"=w549) -> ()  [unwired: 8 in, 2 out]
                            }
                            frame "TEMP" {
                              w556 = 0 items=["FastSettle", "NoOvershoot"] ("Approach")
                              n390 = call "SetTemperature.vi"("Approach"=w556, "Rate"=w554, "Temperature"=w553, "Instrument Ref In"=w555) -> ()  [unwired: 3 in, 3 out]
                              n391 = local write "Temperature setpoint"(w553) -> ()
                            }
                            frame "FIELD" {
                              n392 = call "SetField.vi"("Rate"=w559, "Field"=w557, "Instrument Ref In"=w558) -> ()  [unwired: 4 in, 3 out]
                              n393 = local write "Field Setpoint"(w557) -> ()
                            }
                            frame "THETA" {
                              n394 = local write "Theta Setpoint"(w560) -> ()
                              n395 = call "SetPosition.vi"("Speed"=w562, "Position"=w560, "Instrument Ref In"=w561) -> ()  [unwired: 4 in, 3 out]
                            }
                            frame "CURRENT" {
                              n396 = local read "Measurement \nSetup"() -> (w563:u16)
                              n397 = Number To Exponential String(number=w565) -> (E-format string=w564:string)  [unwired: 3 in]
                              n398 = case shown="0, Default" w563 {
                                tunnel: w564 -> [w566 w577]
                                frame 0, Default {
                                n399 = local read "6221 Address"() -> (w568:string)
                                n400 = local write "Current Amplitude"(w566) -> ()
                                n401 = local read "DC Pulse"() -> (w567:bool)
                                n402 = case shown="True" w567 {
                                tunnel: w568 -> [w571 w574]
                                tunnel: w566 -> [w569 w575]
                                frame False {
                                n403 = Concatenate Strings("CURRent ", w569) -> (w570:string)
                                n404 = GPIB Write(0:w571, 1:w570) -> ()  [unwired: 3 in, 2 out]
                                }
                                frame True {
                                n405 = Concatenate Strings("SOUR:WAVE:AMPL " ("string"), w575) -> (w576:string)
                                n406 = GPIB Write(0:w574, 1:w576) -> ()  [unwired: 3 in, 2 out]
                                }
                                }
                                }
                                frame 1 {
                                n407 = local read "6221 Address 2"() -> (w578:string)
                                n408 = local write "Current Amplitude 2"(w577) -> ()
                                n409 = Concatenate Strings("SOUR:WAVE:AMPL " ("string"), w577) -> (w580:string)
                                n410 = GPIB Write(0:w578, 1:w580) -> ()  [unwired: 3 in, 2 out]
                                }
                              }
                            }
                          }
                        }
                        frame #1 {
                          n411 = local read "Seq Line Now"() -> (w581:i32)
                          n412 = Increment(x=w581) -> (x+1=w582:i32)
                          n413 = local write "Seq Line Now"(w582) -> ()
                          n414 = Wait (ms)(milliseconds to wait=u32 3000) -> ()  [unwired: 1 out]
                        }
                      }
                    }
                  }
                  "Command" <- w182
                  "Current Line" <- w183
                  "ENV VAR" <- w180
                  "Parameters" <- w181
                  "Current Line Number" <- w178
                }
              }
              n415 = And(x=w156, y=w155) -> (x .and. y?=w157:bool)
              n416 = Not(x=w157) -> (.not. x?=w161:bool)
            }
          }
          frame #2 {
            n417 = local write "ExecSeq"(FALSE ("ExecSeq")) -> ()
          }
        }
      }
    }
    n418 = local read "STOP Flag"() -> (w140:bool)
  }
  n419 = while {
    tunnel: w4 -> [w585]
    stop <- w586 stop-if-true
    n420 = local read "Measure Flag"() -> (w587:bool)
    n421 = case shown="True" w587 {
      tunnel: w585 -> [_ w590]
      frame False {
        n422 = Wait (ms)(milliseconds to wait=u32 100) -> ()  [unwired: 1 out]
      }
      frame True {
        n423 = stacked-sequence {
          frame #0 {
            n424 = Wait (ms)(milliseconds to wait=u32 500) -> ()  [unwired: 1 out]
            "Measure Blink" <- TRUE ("Initialised")
          }
          frame #1 {
            n425 = local write "Measure Blink"(FALSE ("Measure Blink")) -> ()
            n426 = Wait (ms)(milliseconds to wait=u32 500) -> ()  [unwired: 1 out]
          }
        }
        n427 = local read "Measurement \nSetup"() -> (w589:u16)
        n428 = stacked-sequence {
          seq-local: [w598 _] -> [_ w693]
          seq-local: [w595 _] -> [_ w690]
          seq-local: [w594 _] -> [_ w691]
          seq-local: [w599 _] -> [_ w694]
          seq-local: [w600 _] -> [_ w695]
          seq-local: [w593 _] -> [_ w692]
          seq-local: [w597 _] -> [_ w688]
          seq-local: [w596 _] -> [_ w689]
          tunnel: w590 -> [w592 _]
          tunnel: w589 -> [w591 _]
          frame #0 {
            n429 = stacked-sequence {
              tunnel: w591 -> [_ w624]
              tunnel: [_ w629] -> w597
              tunnel: [_ w628] -> w596
              tunnel: [_ w627] -> w595
              tunnel: [_ w626] -> w594
              tunnel: [_ w625] -> w593
              frame #0 {
                # "If the flag is ON,\nwe wait for 5s to allow\nthe lock-in and current \nsource to settle.\nThen we turn off the flag\nto not do this again.\nThen we proceed to \nmeasurements."
                # "AC Flag is turned ON if\n- AC Current source of turned ON - inside sequence or with \"Measure Device\" button"
                n430 = local read "AC Flag"() -> (w601:bool)
                n431 = case shown="True" w601 {
                  frame False {
                  }
                  frame True {
                    n432 = stacked-sequence {
                      seq-local: [_ w607 _ _] -> [_ _ w617 _]
                      seq-local: [_ w605 _ _] -> [_ _ w615 _]
                      seq-local: [_ w604 _ _] -> [_ _ w614 _]
                      seq-local: [_ w603 _ _] -> [_ _ w613 _]
                      frame #0 {
                        n433 = Wait (ms)(milliseconds to wait=u32 1000) -> ()  [unwired: 1 out]
                      }
                      frame #1 {
                        w606 = "ARNG;\nASCL;" ("data")
                        n434 = local read "SR860 Ch2 Address"() -> (w603:string)
                        n435 = local read "Ch2 Enable"() -> (w604:bool)
                        n436 = local read "Ch1 Enable"() -> (w605:bool)
                        n437 = local read "SR860 Ch1 Address"() -> (w607:string)
                        n438 = case shown="True" w604 {
                          tunnel: w606 -> [_ w610]
                          tunnel: w603 -> [_ w609]
                          frame False {
                          }
                          frame True {
                            n439 = GPIB Write(0:w609, 1:w610) -> ()  [unwired: 3 in, 2 out]
                          }
                        }
                        n440 = case shown="True" w605 {
                          tunnel: w606 -> [_ w612]
                          tunnel: w607 -> [_ w611]
                          frame False {
                          }
                          frame True {
                            n441 = GPIB Write(0:w611, 1:w612) -> ()  [unwired: 3 in, 2 out]
                          }
                        }
                        n442 = Wait (ms)(milliseconds to wait=u32 1500) -> ()  [unwired: 1 out]
                      }
                      frame #2 {
                        w616 = "APHS;" ("data")
                        n443 = case shown="True" w614 {
                          tunnel: w616 -> [_ w620]
                          tunnel: w613 -> [_ w619]
                          frame False {
                          }
                          frame True {
                            n444 = GPIB Write(0:w619, 1:w620) -> ()  [unwired: 3 in, 2 out]
                          }
                        }
                        n445 = case shown="True" w615 {
                          tunnel: w617 -> [_ w622]
                          tunnel: w616 -> [_ w621]
                          frame False {
                          }
                          frame True {
                            n446 = GPIB Write(0:w622, 1:w621) -> ()  [unwired: 3 in, 2 out]
                          }
                        }
                        n447 = Wait (ms)(milliseconds to wait=u32 3500) -> ()  [unwired: 1 out]
                      }
                      frame #3 {
                        n448 = local write "AC Flag"(FALSE ("AC Flag")) -> ()
                      }
                    }
                  }
                }
              }
              frame #1 {
                n449 = case shown="0, Default" w624 {
                  tunnel: [w643 w666] -> w629
                  tunnel: [w642 w667] -> w628
                  tunnel: [w641 w668] -> w627
                  tunnel: [w640 w669] -> w626
                  tunnel: [w631 w674] -> w625
                  frame 0, Default {
                    # "DC System"
                    n450 = local read "Voltmeter 2 Address"() -> (w633:string)
                    n451 = local read "Voltmeter 1 Address"() -> (w634:string)
                    n452 = local read "Current Amplitude"() -> (w632:string)
                    n453 = local read "Time Period (s)"() -> (w636:string)
                    n454 = local read "6221 Address"() -> (w635:string)
                    n455 = local read "Channel 1"() -> (w638:bool)
                    n456 = local read "Channel 2"() -> (w639:bool)
                    n457 = local read "Tpad(ms)"() -> (w637:i32)
                    n458 = local read "DC Pulse"() -> (w630:bool)
                    n459 = case shown="True" w630 {
                      tunnel: [w653 w665] -> w643
                      tunnel: [w652 w664] -> w642
                      tunnel: [w651 w663] -> w641
                      tunnel: [w650 w662] -> w640
                      tunnel: w639 -> [w644 w661]
                      tunnel: w638 -> [w645 w660]
                      tunnel: w637 -> [_ w659]
                      tunnel: w636 -> [w646 w658]
                      tunnel: w635 -> [_ w657]
                      tunnel: w634 -> [w648 w656]
                      tunnel: w633 -> [w649 w655]
                      tunnel: w632 -> [w647 w654]
                      frame False {
                        n460 = call "DC Basic Measure.vi"("Channel 2"=w644, "Voltmeter 2 Address"=w649, "Channel 1"=w645, "Voltmeter 1 Address"=w648, "Period (s)"=w646, "Amplitude (A)"=w647) -> ("STD 2"=w650:dbl, "Resistance 2"=w651:dbl, "STD 1"=w652:dbl, "Resistance 1"=w653:dbl)  [unwired: 2 in]
                      }
                      frame True {
                        n461 = call "DC Transport Measure.vi"("Channel 2"=w661, "Voltmeter 2 Address"=w655, "Channel 1"=w660, "Voltmeter 1 Address"=w656, "tpad"=w659, "Period (s)"=w658, "Amplitude (A)"=w654, "6221 Address"=w657) -> ("STD 2"=w662:dbl, "Resistance 2"=w663:dbl, "STD 1"=w664:dbl, "Resistance 1"=w665:dbl)
                      }
                    }
                    n462 = Fract/Exp String To Number(string=w632) -> (number=w631:dbl)  [unwired: 3 in, 1 out]
                  }
                  frame 1 {
                    # "AC System"
                    n463 = local read "Buffer Offset (kb)"() -> (w678:string)
                    n464 = local read "Buffer Size (kB)"() -> (w677:i32)
                    n465 = local read "Ch1 Enable"() -> (w679:bool)
                    n466 = local read "Ch2 Enable"() -> (w676:bool)
                    n467 = local read "SR860 Ch1 Address"() -> (w680:string)
                    n468 = local read "SR860 Ch2 Address"() -> (w675:string)
                    n469 = local read "Current Amplitude 2"() -> (w681:string)
                    n470 = Fract/Exp String To Number(string=w681) -> (number=w674:dbl)  [unwired: 3 in, 1 out]
                    n471 = call "AC Transport Measure.vi"("SR860 Ch1 Address"=w680, "Ch1 Enable"=w679, "Buffer Offset (kb)"=w678, "Buffer Size (kb)"=w677, "Ch2 Enable"=w676, "SR860 Ch2 Address"=w675) -> ("R1 Mean"=w673:dbl, "R2 Mean"=w671:dbl, "R1 STD"=w672:dbl, "R2 STD"=w670:dbl)  [unwired: 6 in, 4 out]
                    n472 = Divide(x=w673, y=w674) -> (x/y=w666:dbl)
                    n473 = Divide(x=w672, y=w674) -> (x/y=w667:dbl)
                    n474 = Divide(x=w671, y=w674) -> (x/y=w668:dbl)
                    n475 = Divide(x=w670, y=w674) -> (x/y=w669:dbl)
                  }
                }
              }
            }
            n476 = stacked-sequence {
              tunnel: [_ w686] -> w600
              tunnel: [_ w685] -> w599
              tunnel: [_ w684] -> w598
              tunnel: w592 -> [_ w683]
              frame #0 {
                n477 = Wait (ms)(milliseconds to wait=u32 500) -> ()  [unwired: 1 out]
              }
              frame #1 {
                # "Get PPMS Status\nin the middle of the \ntransport measurement"
                n478 = call "Get All Status.vi"("Instrument Ref In"=w683) -> ("Field"=w685:dbl, "Temperature"=w686:dbl, "Position"=w684:dbl)  [unwired: 3 in, 5 out]
              }
            }
          }
          frame #1 {
            # "Check measure flag before accumulating data as measure flag might've been turned off during the measurement period\nSuch a measurement is often garbage"
            n479 = local read "Serial Number"() -> (w700:i32)
            n480 = local read "Current StartTime"() -> (w696:timestamp)
            n481 = local read "Current Filename"() -> (w698:path)
            n482 = local read "Measure Flag"() -> (w687:bool)
            n483 = Add(x=w700, y=1) -> (x+y=w697:i32)
            n484 = local write "Serial Number"(w697) -> ()
            n485 = case shown="True" w687 {
              tunnel: w698 -> [_ w714]
              tunnel: w697 -> [_ w713]
              tunnel: w696 -> [_ w712]
              tunnel: w695 -> [_ w711]
              tunnel: w694 -> [_ w710]
              tunnel: w693 -> [_ w709]
              tunnel: w692 -> [_ w706]
              tunnel: w691 -> [_ w705]
              tunnel: w690 -> [_ w704]
              tunnel: w689 -> [_ w703]
              tunnel: w688 -> [_ w702]
              frame False {
              }
              frame True {
                n486 = local read "ExecSeq"() -> (w701:bool)
                n487 = case shown="True" w701 {
                  tunnel: w714 -> [_ w743]
                  tunnel: w713 -> [w731 w742]
                  tunnel: w712 -> [w730 w741]
                  tunnel: w711 -> [w728 w740]
                  tunnel: w710 -> [w727 w739]
                  tunnel: w709 -> [w726 w738]
                  tunnel: [w725 w737] -> w708
                  tunnel: w706 -> [w724 w736]
                  tunnel: w705 -> [w720 w735]
                  tunnel: w704 -> [w721 w734]
                  tunnel: w703 -> [w722 w733]
                  tunnel: w702 -> [w723 w732]
                  frame False {
                    n488 = Get Date/Time In Seconds() -> (seconds since 1Jan1904=w719:timestamp)
                    n489 = Subtract(x=w719, y=w730) -> (x-y=w729:dbl)
                    n490 = Build Array(w731, w729, w728, w727, w726, w724, w723, w722, w721, w720) -> (w725:dbl[])
                  }
                  frame True {
                    n491 = call "Create Datafile Entry.vi"("Serial Number"=w742, "Resistance 1"=w732, "STD 1"=w733, "File Name"=w743, "Start time"=w741, "Temperature"=w740, "Field"=w739, "Theta"=w738, "Resistance 2"=w734, "STD 2"=w735, "Current Level"=w736) -> ("Datapoint Array"=w737:dbl[])  [unwired: 3 in, 1 out]
                  }
                }
                n492 = Reshape Array(w708, 1 ("dimension size"), 10 ("dimension size")) -> (w707:dbl[][])
                n493 = local read "Data array"() -> (w716:dbl[][])
                n494 = Insert Into Array(array=w716, new element=w707) -> (w715:dbl[][])  [unwired: 2 in]
                n495 = local write "Data array"(w715) -> ()
              }
            }
          }
        }
      }
    }
    n496 = local read "STOP Flag"() -> (w586:bool)
  }
  "Initialised" <- FALSE ("Initialised")
  "Measure Flag" <- FALSE ("Measure Flag")
  "ExecSeq" <- FALSE ("Initialised")
  "STOP Flag" <- FALSE ("Initialised")
  "AC Flag" <- FALSE ("AC Current Flag")
  "scan_new" <- TRUE ("scan_new")
